vi "DepthProfiling_3D_Core.vi"(5 "BioMAP file path":path=path "", 7 "Params.":variant, 8 "error in (no error)":errorcluster, 9 "Dynamic Params queue":refnum<queue>, 10 "Quit_UserEvent":refnum<user-event>, 11 "ControlQueueRef":variant) -> (0 "error out":errorcluster, 2 "Output":variant)   [LabVIEW 2013]
uses:
  Apps_static/ScanParams_SingleLine.ctl
  ProcessMethods/Binning/BinType.ctl
  Files/BinaryHeader.ctl
  ControlDef/QueueRefs.ctl
  ControlDef/LaserCtrl_Method.ctl
  ControlDef/States-AToF.ctl
  <instrlib>/AnalogDiscSDKLv/VIs/DWF_CtrlQueue.ctl
  <instrlib>/AnalogDiscSDKLv/VIs/DWF_State.ctl
  <instrlib>/ESP300/Public/Data/ESP300_State.ctl
  <instrlib>/DG535/Command/DG535_States.ctl
  Hardware/BNC(QuantumComposers)/BNC_States.ctl
  Hardware/FemtoLaser(Legacy)/Laser_Status.ctl
  Hardware/DAQmx(Legacy)/DAQmx_Status.ctl
  ControlDef/Signal.ctl
  ProcessMethods/SignalAverager/ProcessStates.ctl
  Files/WriterState.ctl
  Files/Signal_Segment.ctl
  ControlDef/ProcessingMode.ctl
  Hardware/EPM2000(Legacy)/EPM2K_Status.ctl
  <instrlib>/AnalogDiscSDKLv/VIs/DWF_Signal.ctl
  ControlDef/SampleRateSelector.ctl
  ImagingMS/DirectImaging_State.ctl
  ImagingMS/Imaging_Params.ctl
  ProcessMethods/BioMapConversion/BioMAPWriterCoreParams.ctl
  <vilib>/Utility/error.llb/DialogType.ctl
  <vilib>/Utility/miscctls.llb/LVRowAndColumnTypeDef.ctl
  <vilib>/picture/picture.llb/imagedata.ctl
  <vilib>/Analysis/baseanly.llb/Mean (DBL).vi
  UI/Autoscale_Y_Single.vi
  <userlib>/_OpenG.lib/comparison/comparison.llb/I32 Changed__ogtk.vi
  ProcessMethods/Binning/SpectrumBinning.vi
  <vilib>/regexp/Match Regular Expression.xnode
  <instrlib>/ESP300/ESP300.lvlib
  <instrlib>/DG535/SRS_DG535_Lib.lvlib
  <userlib>/Utility/ErrorLog_lib.lvlib
  <instrlib>/AnalogDiscSDKLv/AnalogDiscSDKLv.lvlib
  <vilib>/Analysis/NI_AALBase.lvlib
panel:
  out "m/z":dbl=11.0
  in  "Linear/Log":bool
  in  "Integration Width (±Da)":dbl=0.5
  in  "m/z (Da)":dbl=11.0
  in  "BinType":T1=enum."ByMass"
  in  "BinWidth":dbl=0.2 min=0.001
  in  "#Layers":i32=1 caption="LayerAverage#" min=1 max=2000 step=1
  in  "Shot#":i32=1 caption="nth of Shot" min=1 max=65535 step=1
  in  "X--":bool
  in  "X++":bool
  in  "Fullscale X":bool
  in  "Fullscale Y":bool
  in  "Y--":bool
  in  "Y++":bool
  out "Depth Profile":dbl[](graph)
  out "Spectra":cluster{"Array":dbl[], dbl[]}(graph)
  in  "MaxiMass":dbl=300.0 format="%#_13g"
  in  "EnableBinning":bool
  out "Information":string
  in  "AutoScaleZ":bool
  in  "SaveMiddleFile":bool
  in  "Color Scheme":T2(ring)=enum."Rainbow"
  out "#SOL":i32
  out "#EOL":i32
  out "remaining lines":i32
  out "State":T3(ring)
  out "Line#":i32
  in  "Cancel":bool
  in  "Close/Quit":bool
  in  "Peaks of Interest":string[][](table)=[["300", "300"], ["68", ".45"], ["92", ".45"], ["114", ".45"]]
  in  "conv. coeff.":sgl=6553.0
  out "# average":i32
  in  "Start":bool
  out "ImagePreview":dbl[][](graph)
  in  "PeakOI #":i32
  out "MS (Raw)":cluster{"m/z_Array":dbl[], sgl[]}(graph)
  out "Iteration":i32
  out "Export File Path":path caption="Filename"
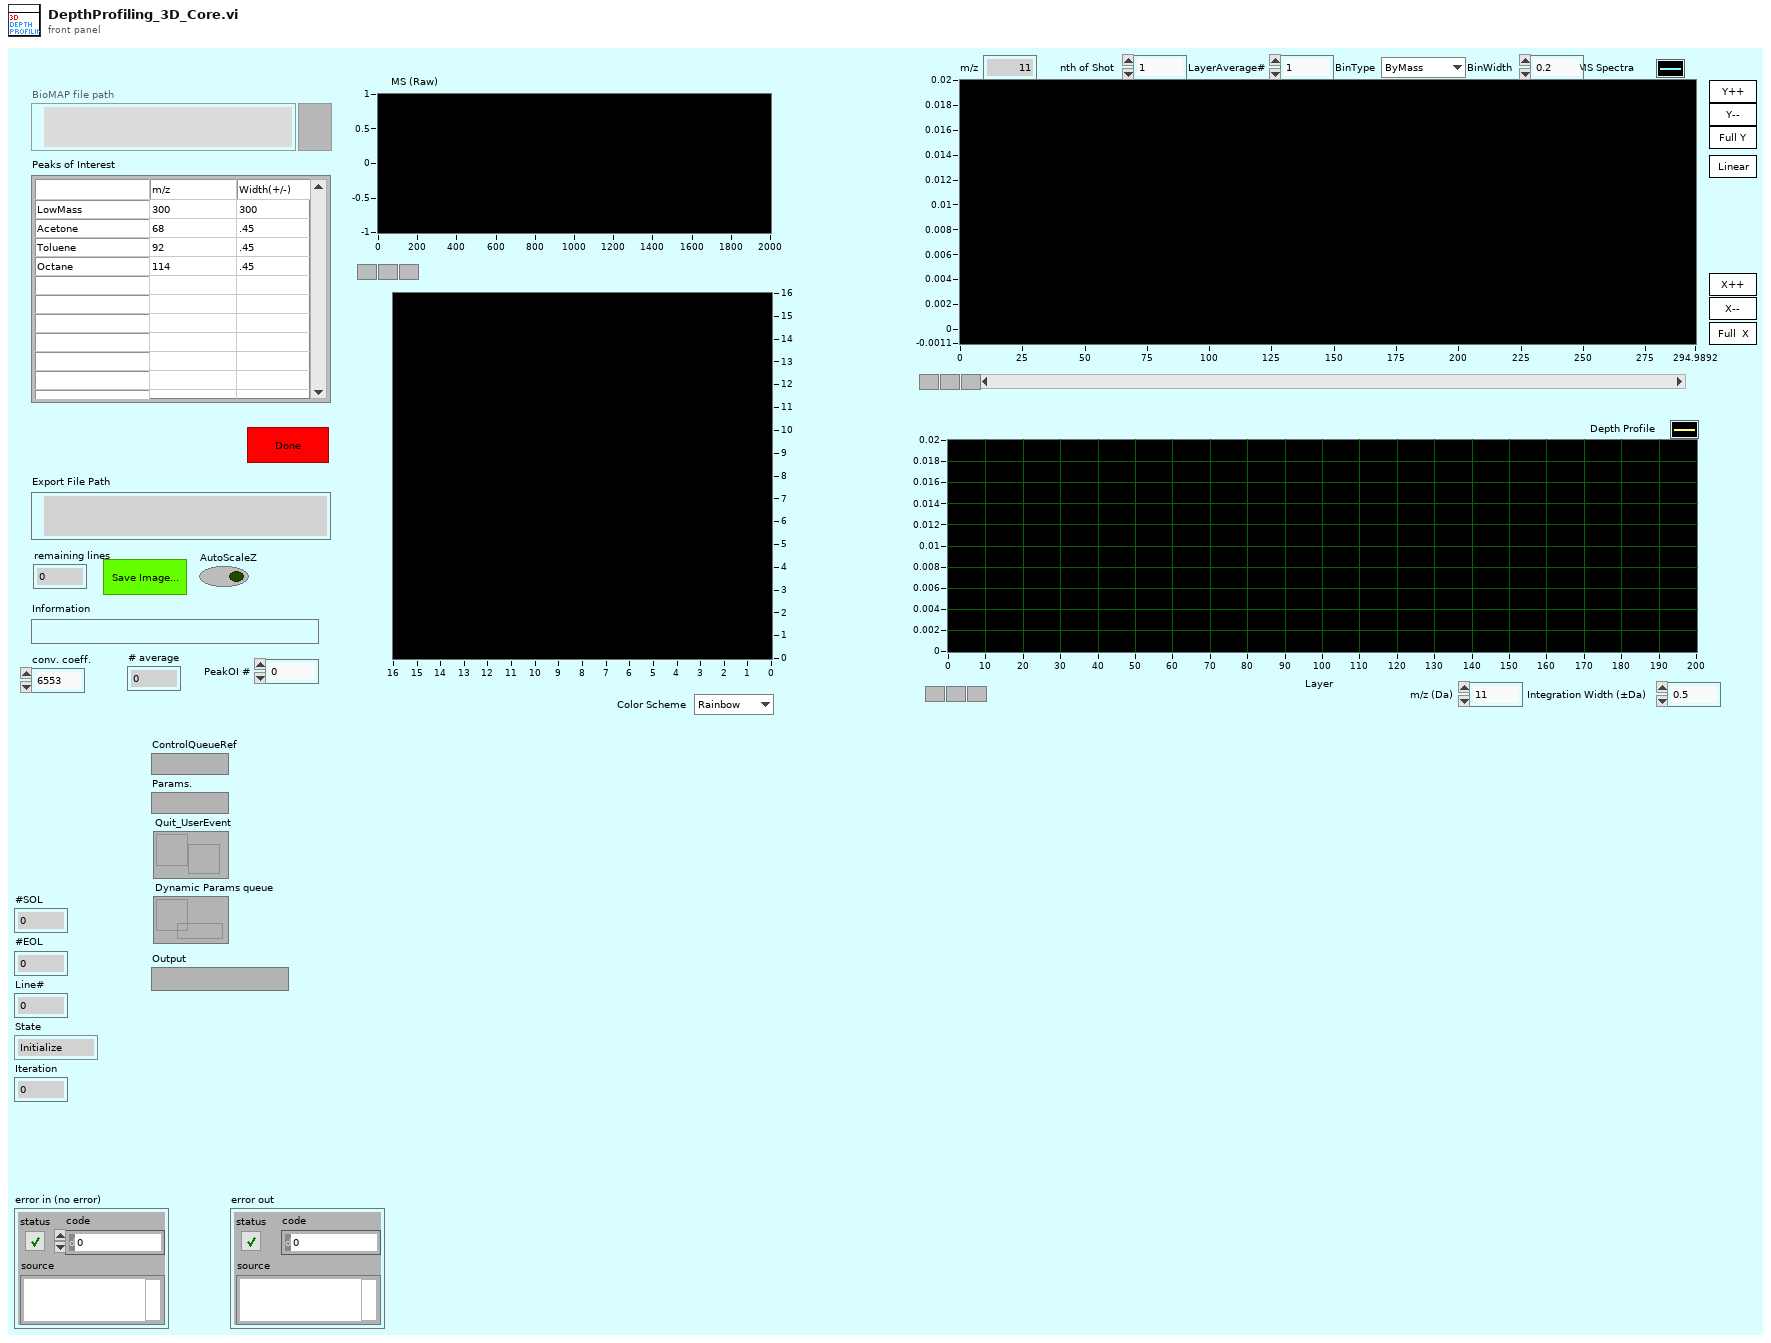
[diagram p1: front panel]
types:
  T1 = typedef "BinType.ctl" = enum16{"ByTime", "ByScreen", "ByMass", "ToUnitMass"}
  T2 = enum16{"Greyscale", "Rainbow", "Jet", "Rainbow_Wh", "Banded", "Seis", "InvertSeis", "Jaisnd", "TBD1"}
  T3 = enum16{"Initialize", "Open", "PrepScanParams", "WaitData", "Flush", "ScanResult", "CheckEndCondition", "Close", "Quit", "Refresh_Image", "Refresh_Profile", "Refresh_Spectra", "Refresh_RawSpectrum", "SaveMiddleFile", "Save_Image", "SetPeakOI"}
  T4 = cluster{"image path":path, "file refnum":refnum<file>}
  T5 = enum8{"Enabled", "Disabled", "Disabled and Grayed Out"}
  T6 = typedef "QueueRefs.ctl" = cluster{"LaserCtrlMethod":T7, "Apps":refnum<queue>, "MainDAQCoreQueue":refnum<queue>, "Micos":refnum<queue>, "ESP300":refnum<queue>, "SMC100":refnum<queue>, "SRS DG535":refnum<queue>, "BNC":refnum<queue>, "SDG_ii":refnum<queue>, "NI-USB_DAQmx":refnum<queue>, "ProcCore_CtrlQueue":refnum<queue>, "WriterCtrl":refnum<queue>, "WriterSIG":refnum<queue>, "Feedback":refnum<queue>, "EPM2000":refnum<queue>, "InfoRef":refnum<vi>, "AppsLock":T8, "ProcCore_SignalQueue":refnum<queue>}
  T7 = typedef "LaserCtrl_Method.ctl" = enum16{"SRS_DG535", "BNC", "SDG_II"}
  T8 = typedef "Semaphore RefNum" = refnum<k1>
  T9 = typedef "ProcessStates.ctl" = enum16{"Initialize", "Normal", "Display", "Write2Buffer", "CalcMzArray", "StartSave", "StopSave", "ConfigChanged", "EndOfLine", "SetFilterParams", "SetGraphsEnable", "SetAcquisitionParams", "ChangeDisplayIncrement", "ChangeRepRate", "SetWriterRef", "Quit", "StartOfLine"}
  T10 = cluster{"Average":i32, "X (Img)":i32, "Y (Img)":i32, "Spectra":sgl[], "Depth":i32, "TickCount":dbl}
  T11 = typedef "BioMAPWriterCoreParams.ctl" = cluster{"File Header":T12, "mzCali.":dbl[], "m/z_Array":dbl[], "SampleRate":T13, "TrigDelay":dbl, "file refnum":refnum<file>, "file path":path, "PeakOI":cluster{"m/z":dbl, "Width(+/-)":dbl}[], "Binning":cluster{"Enable":bool, "BinType":T1, "BinWidth":dbl, "Maximum":dbl, "Minimum":dbl}}
  T12 = typedef "BinaryHeader.ctl" = cluster{"Start Position":dbl[], "StepWidth":dbl[], "Dimension":i32[], "SpecLength":i32}
  T13 = typedef "SampleRateSelector.ctl" = dbl
  T14 = typedef "Imaging_Params.ctl" = cluster{"File Header":T12, "ScanSpeed":dbl, "HighSpeed":dbl, "SampleRate":T13, "Rep.Rate (Hz)":dbl, "TrigDelay":dbl, "mzCali":dbl[], "KeepStill(ms)":u32, "SaveRaw":bool}
  T15 = typedef "DirectImaging_State.ctl" = cluster{"State":enum16{"Initialize", "Open", "PrepScanParams", "WaitData", "Flush", "ScanResult", "CheckEndCondition", "Close", "Quit", "Refresh_Image", "Refresh_Profile", "Refresh_Spectra", "Refresh_RawSpectrum", "SaveMiddleFile", "Save_Image", "SetPeakOI"}, "Para.":variant}
  T16 = cluster{"Save?":bool, "File Header":T12, "Scan#":i32, "ControlRefs":T6, "HighSpeed":dbl, "ScanSpeed":dbl, "SampleRate":T13, "mzCali.":dbl[], "TrigDelay":dbl, "InfoBarRef.":refnum<vi>, "mzArray":dbl[], "SaveRaw":bool, "RepRate":dbl}
  T17 = typedef "LVRowAndColumnTypeDef.ctl" = cluster{"Row":i32, "Column":i32}
  T18 = typedef "DialogType.ctl" = u16
  T19 = typedef "LVPoint32TypeDef.ctl" = cluster{"Horizontal":i32, "Vertical":i32}
  T20 = typedef "LVRectTypeDef.ctl" = cluster{"Left":i16, "Top":i16, "Right":i16, "Bottom":i16}
  T21 = enum16{"open", "replace", "create", "open or create", "replace or create", "replace or create with confirmation"}
  T22 = cluster{"queue out":refnum<queue>, "queue out":refnum<queue>}
  T23 = typedef "Signal.ctl" = cluster{"Command":T9, "Params":variant}
  T24 = typedef "Signal_Segment.ctl" = cluster{"SampleRate":dbl, "TrigDelay":dbl, "SpecLength":dbl, "DAQ_Range":dbl, "Average#":i32, "Position":dbl[], "Spectrum":sgl[], "Calibr.":dbl[], "Pressure":dbl, "Desp_LaserEnergy":dbl, "PI_LaserEnergy":dbl, "Voltages Table":sgl[][], "ProcMode":T25, "Threshold":dbl, "Comment":string, "TickCount":dbl, "Time Stamp":timestamp}
  T25 = typedef "ProcessingMode.ctl" = enum16{"None", "Drop by Threshold", "TDC Simulate", "SetFilter"}
  T26 = typedef "ScanParams_SingleLine.ctl" = cluster{"Line Start":dbl[], "Line End":dbl[], "HighSpeed":dbl, "ScanSpeed":dbl, "KeepStill(ms)":u32, "InstruParams":dbl[]}
  T27 = typedef "imagedata.ctl" = cluster{"image type":i32, "image depth":i32, "image":u8[], "mask":u8[], "colors":u32[], "Rectangle":cluster{"left":i16, "top":i16, "right":i16, "bottom":i16}}
  T28 = cluster{"Rows Per Strip":i32, "Photometric":i32, "Compression Type":i32}
  T29 = cluster{"Average":i32, "X (Img)":i32, "Y (Img)":i32, "Spectra":sgl[], "Depth":i32, "TickCount":dbl}[]
  T30 = typedef "IMAQ Image.ctl" = refnum<image>
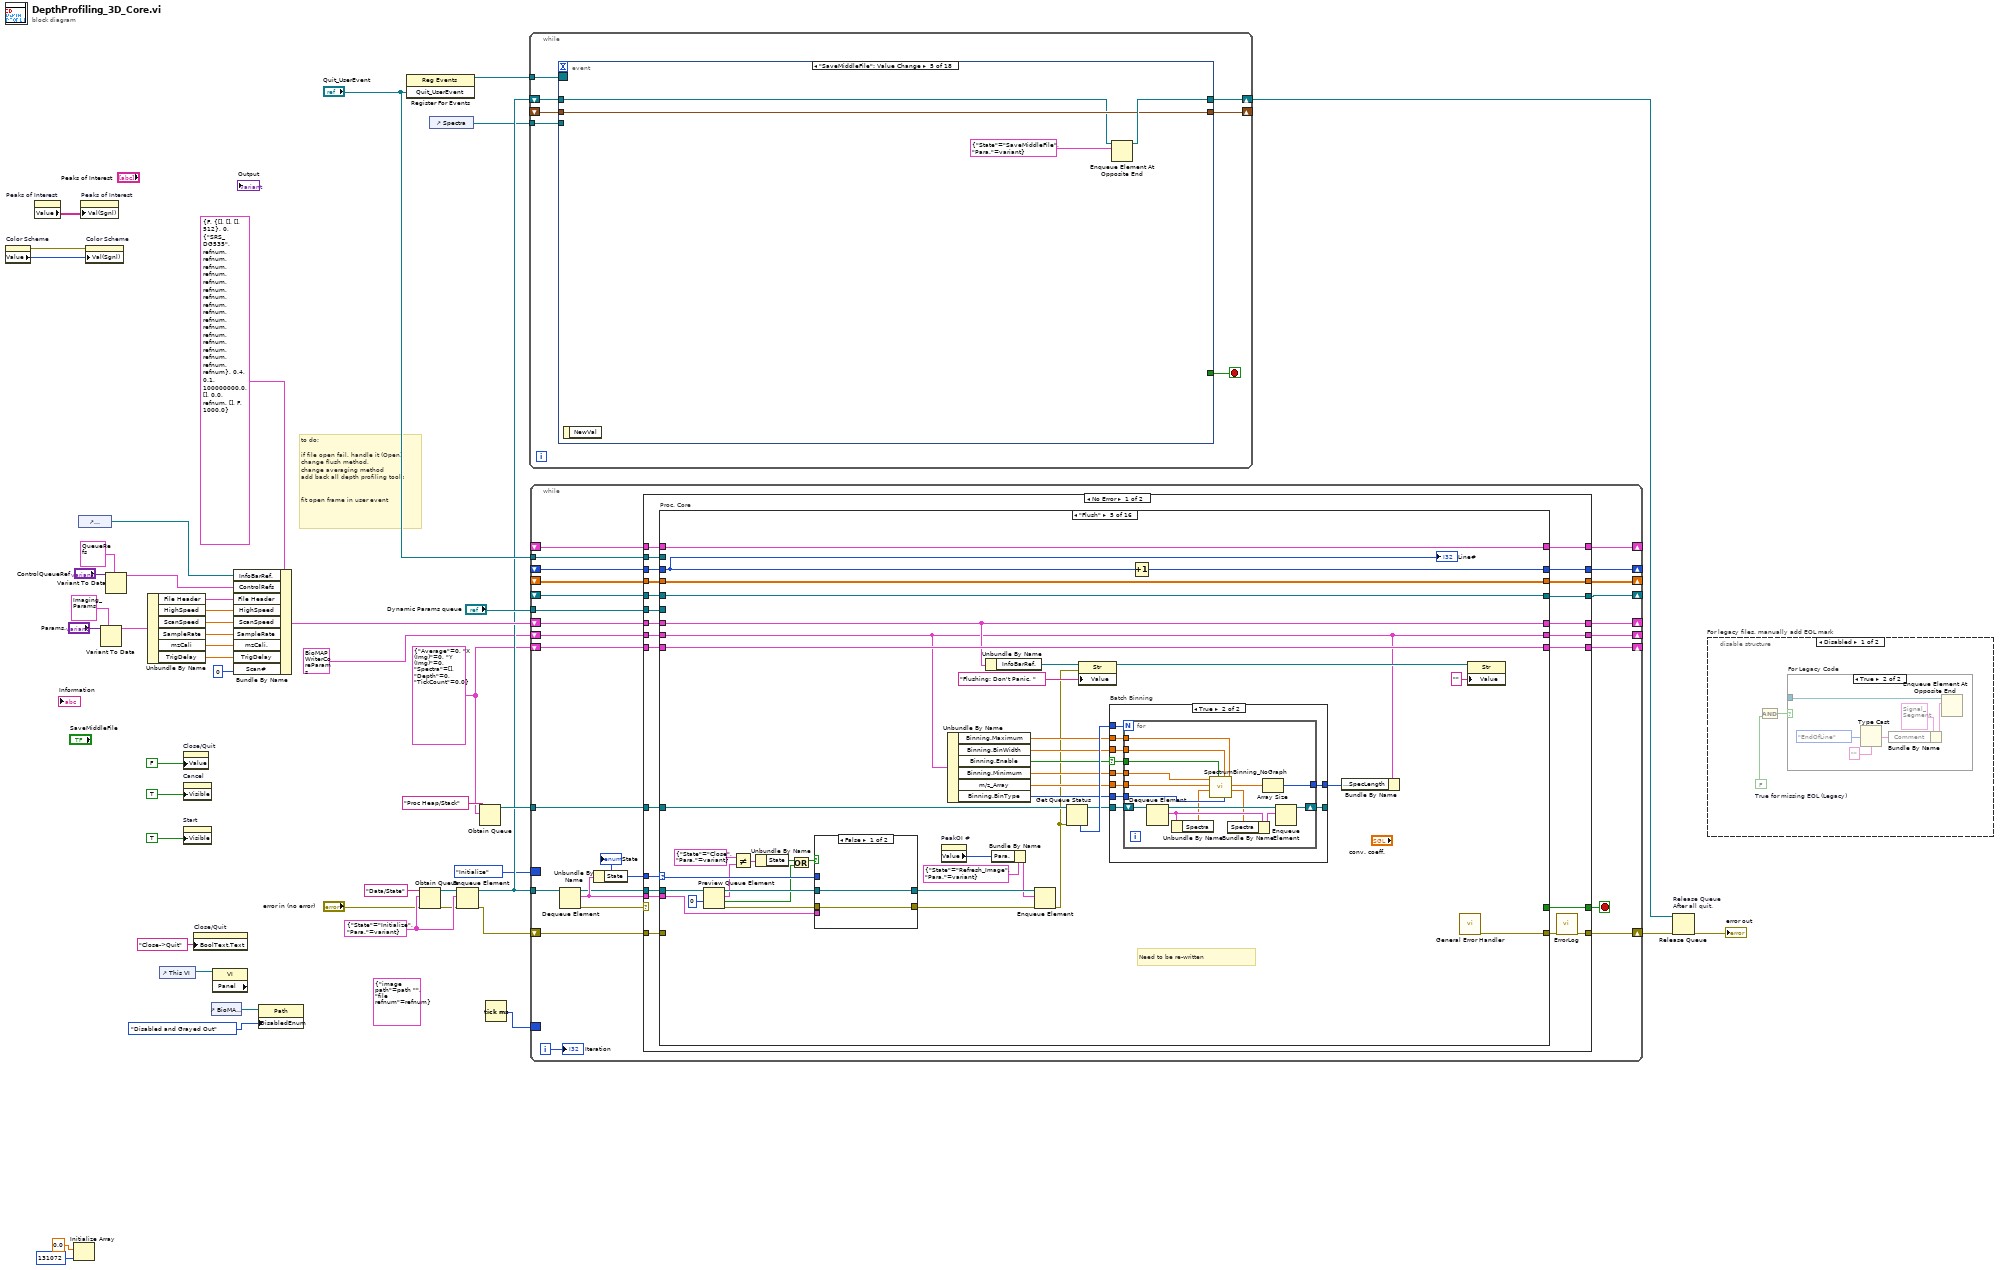
[diagram p0: block diagram]
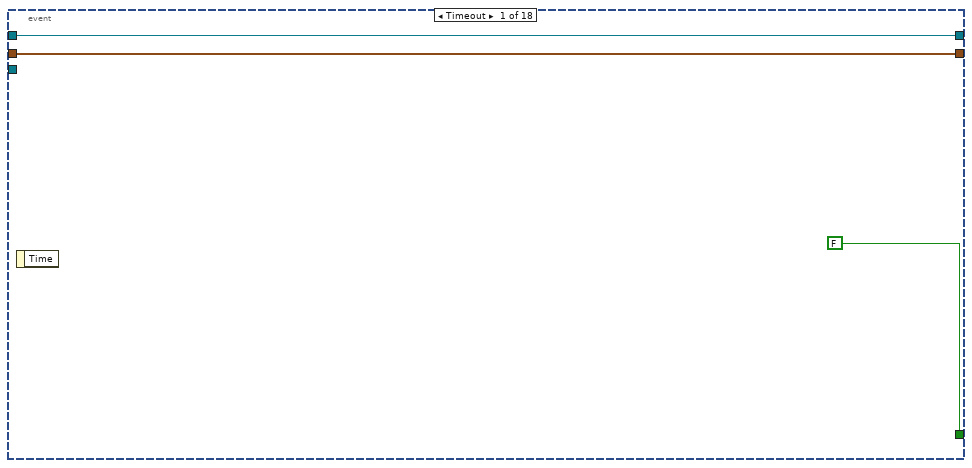
[diagram p4: hidden frame]
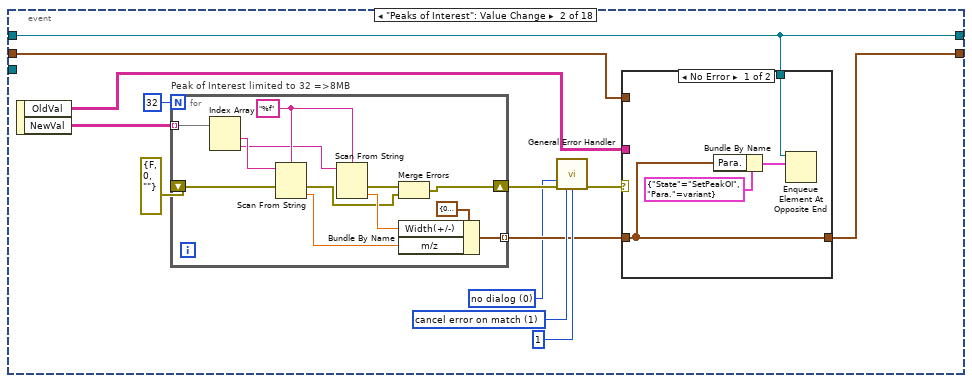
[diagram p5: hidden frame]
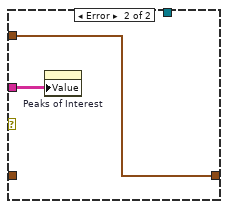
[diagram p6: hidden frame]
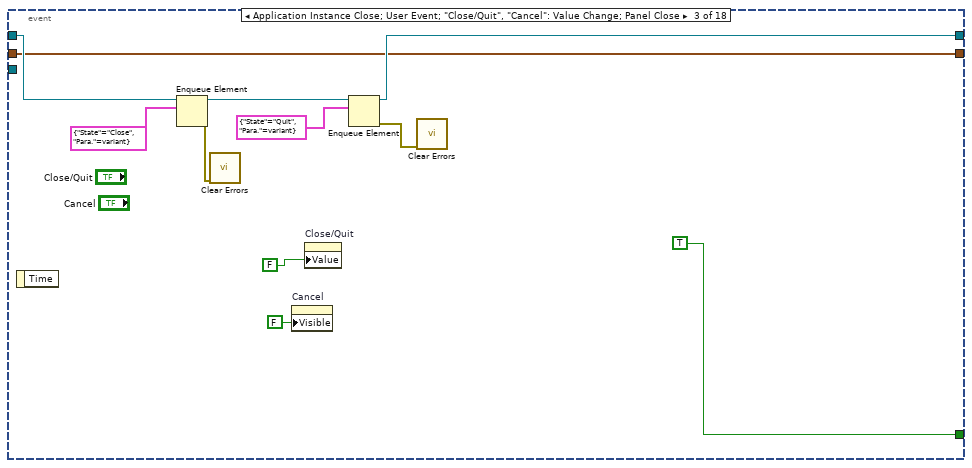
[diagram p7: hidden frame]
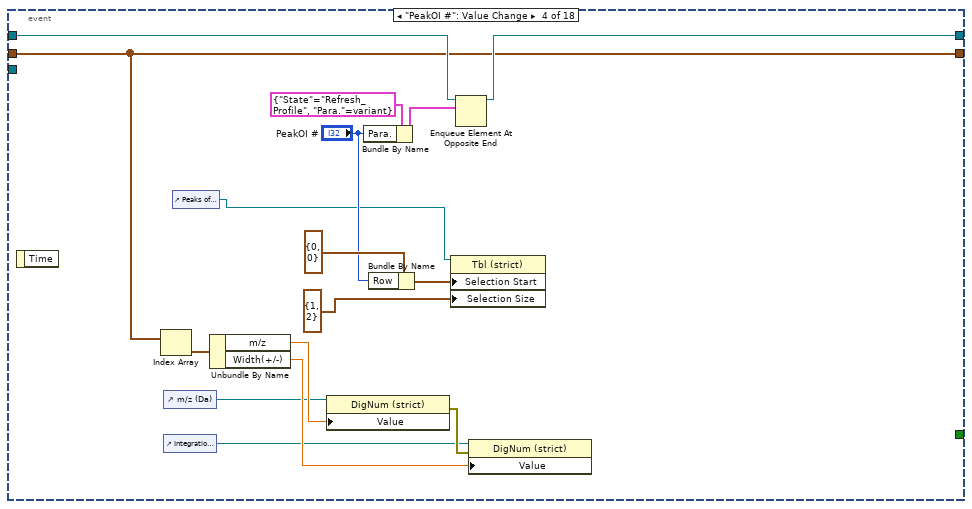
[diagram p8: hidden frame]
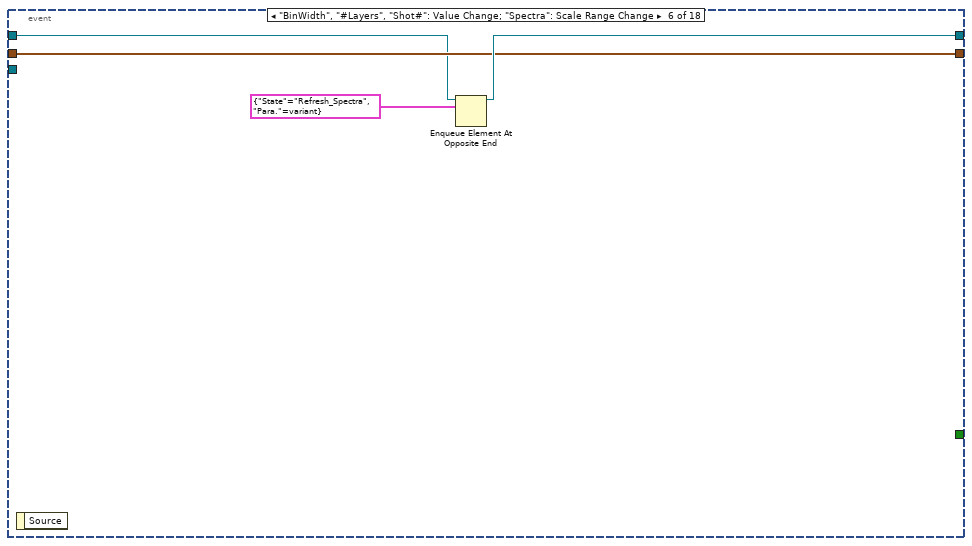
[diagram p9: hidden frame]
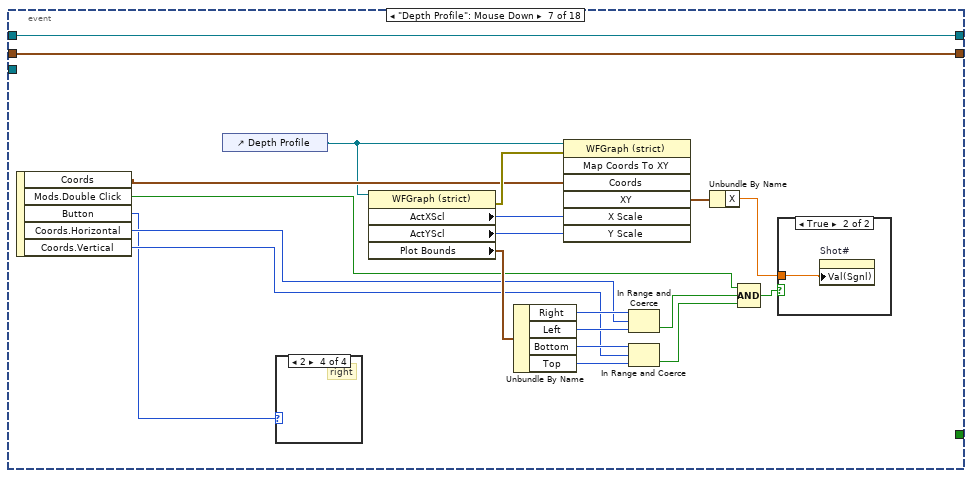
[diagram p10: hidden frame]
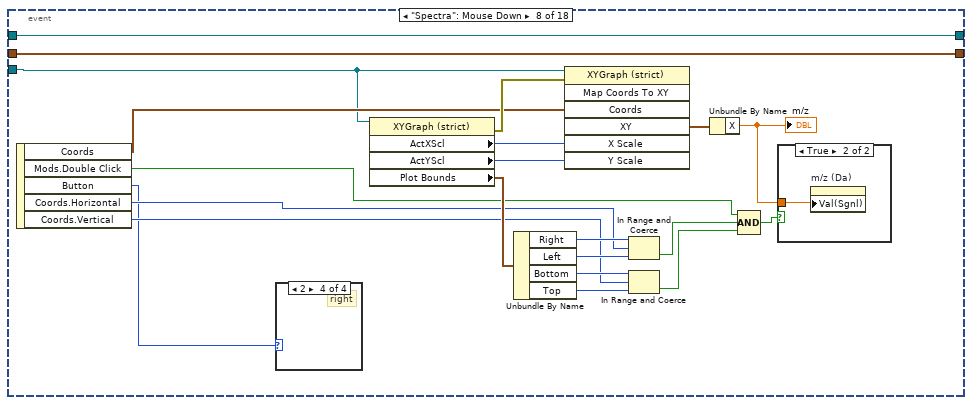
[diagram p15: hidden frame]
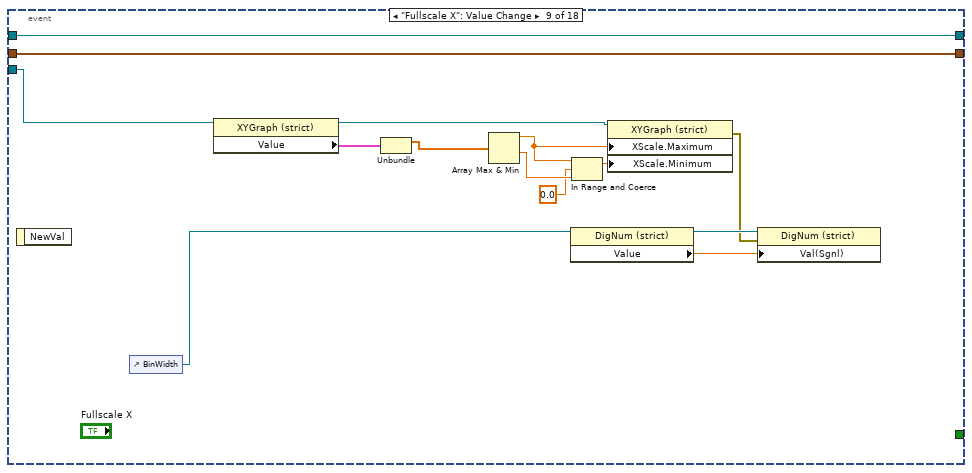
[diagram p20: hidden frame]
diagram:
  (unwired) T4 {"image path"=path "", "file refnum"=refnum} ("output cluster")
  w26 = T10 {"Average"=0, "X (Img)"=0, "Y (Img)"=0, "Spectra"=[], "Depth"=0, "TickCount"=0.0} ("output cluster")
  w38 = T15 {"State"=enum."Initialize", "Para."=variant}
  # "to do;\n\nif file open fail, handle it (Open)\nchange flush method,\nchange averaging method\nadd back all depth profiling tools\n\n\nfit open frame in user event"
  n1 = property on="Color Scheme" class="Enum (strict)"() -> (error out=w2:errorcluster, "Value"=w3:T2)  [unwired: 2 in, 1 out]
  n2 = property on="Peaks of Interest" class="Tbl (strict)"() -> ("Value"=w7:string[][])  [unwired: 2 in, 2 out]
  n3 = Initialize Array(sgl 0.0 ("element"), 131072 ("dimension size")) -> ()  [unwired: 1 out]
  n4 = control-ref of="Information"() -> (w5:refnum<vi>)
  n5 = property on="Peaks of Interest" class="Tbl (strict)"("Val(Sgnl)"=w7) -> ()  [unwired: 2 in, 2 out]
  n6 = property on="Color Scheme" class="Enum (strict)"(error in=w2, "Val(Sgnl)"=w3) -> ()  [unwired: 1 in, 2 out]
  n7 = Variant To Data(type=T14 {"File Header"={"Start Position"=[], "StepWidth"=[], "Dimension"=[], "SpecLength"=0}, "ScanSpeed"=0.0, "HighSpeed"=0.0, "SampleRate"=0.0, "Rep.Rate (Hz)"=0.0, "TrigDelay"=0.0, "mzCali"=[], "KeepStill(ms)"=0, "SaveRaw"=FALSE} ("BeamProfiling_Params"), Variant="Params.") -> (data=w33:T14)  [unwired: 1 in, 1 out]
  n8 = Variant To Data(type=T6 {"LaserCtrlMethod"=enum."SRS_DG535", "Apps"=refnum, "MainDAQCoreQueue"=refnum, "Micos"=refnum, "ESP300"=refnum, "SMC100"=refnum, "SRS DG535"=refnum, "BNC"=refnum, "SDG_ii"=refnum, "NI-USB_DAQmx"=refnum, "ProcCore_CtrlQueue"=refnum, "WriterCtrl"=refnum, "WriterSIG"=refnum, "Feedback"=refnum, "EPM2000"=refnum, "InfoRef"=refnum, "AppsLock"=refnum, "ProcCore_SignalQueue"=refnum} ("ControlRefs"), Variant="ControlQueueRef") -> (data=w13:T6)  [unwired: 1 in, 1 out]
  n9 = Unbundle By Name(w33) -> ("File Header"=w32:T12, "HighSpeed"=w31:dbl, "ScanSpeed"=w30:dbl, "SampleRate"=w28:T13, "mzCali"=w19:dbl[], "TrigDelay"=w18:dbl)
  n10 = control-ref of="This VI"() -> (w17:refnum<vi>)
  n11 = property on="Close/Quit" class="Bool (strict)"("Value"=FALSE) -> ()  [unwired: 2 in, 2 out]
  n12 = property on="Cancel" class="Bool"("Visible"=TRUE) -> ()  [unwired: 2 in, 2 out]
  n13 = property on="Start" class="Bool"("Visible"=TRUE) -> ()  [unwired: 2 in, 2 out]
  n14 = property on="Close/Quit" class="Bool (strict)"("BoolText.Text"="Close->Quit" ("Boolean Text.Text")) -> ()  [unwired: 2 in, 2 out]
  n15 = control-ref of="BioMAP file path"() -> (w12:refnum<vi>)
  n16 = property class="VI" props=["Panel"](reference=w17) -> ()  [unwired: 1 in, 3 out]
  n17 = Bundle By Name(cluster=T16 {"Save?"=FALSE, "File Header"={"Start Position"=[], "StepWidth"=[], "Dimension"=[], "SpecLength"=512}, "Scan#"=0, "ControlRefs"={"LaserCtrlMethod"=enum."SRS_DG535", "Apps"=refnum, "MainDAQCoreQueue"=refnum, "Micos"=refnum, "ESP300"=refnum, "SMC100"=refnum, "SRS DG535"=refnum, "BNC"=refnum, "SDG_ii"=refnum, "NI-USB_DAQmx"=refnum, "ProcCore_CtrlQueue"=refnum, "WriterCtrl"=refnum, "WriterSIG"=refnum, "Feedback"=refnum, "EPM2000"=refnum, "InfoRef"=refnum, "AppsLock"=refnum, "ProcCore_SignalQueue"=refnum}, "HighSpeed"=0.4, "ScanSpeed"=0.1, "SampleRate"=100000000.0, "mzCali."=[], "TrigDelay"=0.0, "InfoBarRef."=refnum, "mzArray"=[], "SaveRaw"=FALSE, "RepRate"=1000.0} ("output cluster"), "InfoBarRef."=w5, "ControlRefs"=w13, "File Header"=w32, "HighSpeed"=w31, "ScanSpeed"=w30, "SampleRate"=w28, "mzCali."=w19, "TrigDelay"=w18, "Scan#"=0) -> (w42:T16)
  n18 = property class="Path"(reference=w12, "DisabledEnum"=T5."Disabled and Grayed Out" ("Disabled")) -> ()  [unwired: 1 in, 2 out]
  n19 = register-events("Quit_UserEvent") -> (reference out=w43:refnum<event-registration>)  [unwired: 2 in, 1 out]
  n20 = Obtain Queue(name (unnamed)="Data/State", element data type=w38, error in (no error)="error in (no error)") -> (queue out=w39:refnum<queue>, error out=w37:errorcluster)  [unwired: 2 in, 1 out]
  n21 = control-ref of="Spectra"() -> (w1:refnum<vi>)
  n22 = Enqueue Element(queue=w39, element=w38, error in (no error)=w37) -> (queue out=w35:refnum<queue>, error out=w27:errorcluster)  [unwired: 1 in, 1 out]
  n23 = Obtain Queue(name (unnamed)="Proc Heap/Stack", element data type=w26) -> (queue out=w48:refnum<queue>)  [unwired: 3 in, 2 out]
  n24 = Tick Count (ms)() -> (millisecond timer value=w25:u32)
  n25 = while {
    tunnel: w43 -> [w53]
    shift-right: [w52] -> w20
    shift-left: w35 -> [w55]
    shift-right: [w51] -> _
    shift-left: _ -> [w50]
    tunnel: w1 -> [w49]
    stop <- w54 stop-if-true
    n26 = event shown="[4] \"SaveMiddleFile\": Value Change" {
      selector: w53 -> [_ _ _ _ _ _ _ _ _ _ _ _ _ _ _ _ _ _]
      dyn-events: _ -> [_ _ _ _ _ _ _ _ _ _ _ _ _ _ _ _ _ _]
      timeout: _ -> [_ _ _ _ _ _ _ _ _ _ _ _ _ _ _ _ _ _]
      tunnel: w55 -> [w57 w59 w97 w113 w117 w121 w145 w167 w182 w185 w192 w210 w228 w250 w279 w290 w313 w345]
      tunnel: [FALSE _ TRUE _ _ _ _ _ _ _ _ _ _ _ _ _ _ _] -> w54
      tunnel: [w57 w59 w93 w114 w119 w123 w145 w167 w182 w185 w192 w210 w228 w250 w279 w290 w308 w344] -> w52
      tunnel: [w56 w64 w92 w104 w118 w122 w144 w166 w181 w184 w191 w209 w227 w249 w278 w287 w310 w343] -> w51
      tunnel: w50 -> [w56 w62 w92 w104 w118 w122 w144 w166 w181 w184 w191 w209 w227 w249 w278 w287 w310 w343]
      tunnel: w49 -> [_ _ _ _ _ _ _ w147 w169 w183 w187 w193 w211 w229 w258 _ _ _]
      event Timeout {
        n27 = event-data() -> ()  [unwired: 1 in, 1 out]
      }
      event "Peaks of Interest": Value Change {
        w60 = T18 0 items=["no dialog", "OK message", "continue or stop message", "OK message + warnings", "continue/stop + warnings"] ("type of dialog (OK msg:1)")
        w65 = 1 items=["no exception", "cancel error on match", "set error on match"] ("[exception action] (none:0)")
        n28 = event-data() -> ("OldVal"=w70:string[][], "NewVal"=w71:string[][])  [unwired: 1 in]
        n29 = for "Peak of Interest limited to 32 =>8MB" {
          N: 32 -> [_]
          tunnel: w71 -> [w83] mode=indexing
          shift-right: [w75] -> w66
          shift-left: errorcluster {"status"=FALSE, "code"=0, "source"=""} ("error IO") -> [w77]
          tunnel: [w76] -> w63 mode=indexing
          w82 = "%f" ("format string")
          n30 = Index Array(array=w83) -> (element #1=w73:string, element #2=w72:string)  [unwired: 2 in]
          n31 = Scan From String(format string=w82, input string=w73, error in=w77) -> (error out=w74:errorcluster, output 1=w79:dbl)  [unwired: 2 in, 2 out]
          n32 = Scan From String(format string=w82, input string=w72) -> (error out=w78:errorcluster, output 1=w80:dbl)  [unwired: 3 in, 2 out]
          n33 = Merge Errors(w78, w74) -> (w75:errorcluster)
          n34 = Bundle By Name(cluster=cluster{"m/z":dbl, "Width(+/-)":dbl} {"m/z"=0.0, "Width(+/-)"=0.0} ("Peak-Of-Interest"), "Width(+/-)"=w80, "m/z"=w79) -> (w76:cluster{"m/z":dbl, "Width(+/-)":dbl})
        }
        n35 = call <vilib>:"General Error Handler.vi"("type of dialog (OK msg:1)"=w60, "error in (no error)"=w66, "[exception action] (none:0)"=w65, "[exception code]"=1) -> ("error out"=w67:errorcluster)  [unwired: 7 in, 4 out]
        n36 = case shown="No Error" w67 {
          tunnel: w70 -> [_ w89]
          tunnel: [w85 w88] -> w64
          tunnel: w63 -> [w85 _]
          tunnel: w62 -> [_ w88]
          tunnel: w59 -> [w84 _]
          frame No Error {
            n37 = Bundle By Name(cluster=T15 {"State"=enum."SetPeakOI", "Para."=variant} ("element"), "Para."=w85) -> (w86:T15)
            n38 = Enqueue Element At Opposite End(queue=w84, element=w86) -> ()  [unwired: 2 in, 3 out]
          }
          frame Error {
            n39 = property on="Peaks of Interest" class="Tbl (strict)"("Value"=w89) -> ()  [unwired: 2 in, 2 out]
          }
        }
      }
      event Application Instance Close; User Event; "Close/Quit", "Cancel": Value Change; Panel Close {
        n40 = event-data() -> ()  [unwired: 1 in, 1 out]
        n41 = Enqueue Element(queue=w97, element=T15 {"State"=enum."Close", "Para."=variant}) -> (queue out=w98:refnum<queue>, error out=w96:errorcluster)  [unwired: 2 in, 1 out]
        n42 = call <vilib>:"Clear Errors.vi"("error in (no error)"=w96) -> ()  [unwired: 6 in, 1 out]
        n43 = property on="Cancel" class="Bool"("Visible"=FALSE) -> ()  [unwired: 2 in, 2 out]
        n44 = property on="Close/Quit" class="Bool (strict)"("Value"=FALSE) -> ()  [unwired: 2 in, 2 out]
        n45 = Enqueue Element(queue=w98, element=T15 {"State"=enum."Quit", "Para."=variant}) -> (queue out=w93:refnum<queue>, error out=w99:errorcluster)  [unwired: 2 in, 1 out]
        n46 = call <vilib>:"Clear Errors.vi"("error in (no error)"=w99) -> ()  [unwired: 6 in, 1 out]
      }
      event "PeakOI #": Value Change {
        n47 = event-data() -> ()  [unwired: 1 in, 1 out]
        n48 = Index Array(array=w104) -> (element=w105:cluster{"m/z":dbl, "Width(+/-)":dbl})  [unwired: 1 in]
        n49 = control-ref of="m/z (Da)"() -> (w102:refnum<vi>)
        n50 = control-ref of="Integration Width (±Da)"() -> (w101:refnum<vi>)
        n51 = control-ref of="Peaks of Interest"() -> (w108:refnum<vi>)
        n52 = Unbundle By Name(w105) -> ("m/z"=w103:dbl, "Width(+/-)"=w106:dbl)
        n53 = property class="DigNum (strict)"(reference=w102, "Value"=w103) -> (error out=w107:errorcluster)  [unwired: 1 in, 1 out]
        n54 = Bundle By Name(cluster=T15 {"State"=enum."Refresh_Profile", "Para."=variant} ("element"), "Para."="PeakOI #") -> (w115:T15)
        n55 = Bundle By Name(cluster=T17 {"Row"=0, "Column"=0} ("Selection Start"), "Row"="PeakOI #") -> (w111:T17)
        n56 = property on="Property Node" class="Tbl (strict)"(reference=w108, "Selection Start"=w111, "Selection Size"=T17 {"Row"=1, "Column"=2}) -> ()  [unwired: 1 in, 2 out]
        n57 = Enqueue Element At Opposite End(queue=w113, element=w115) -> (queue out=w114:refnum<queue>)  [unwired: 2 in, 2 out]
        n58 = property class="DigNum (strict)"(reference=w101, error in=w107, "Value"=w106) -> ()  [unwired: 2 out]
      }
      event "SaveMiddleFile": Value Change {
        n59 = event-data() -> ()  [unwired: 1 in, 1 out]
        n60 = Enqueue Element At Opposite End(queue=w117, element=T15 {"State"=enum."SaveMiddleFile", "Para."=variant}) -> (queue out=w119:refnum<queue>)  [unwired: 2 in, 2 out]
      }
      event "BinWidth", "#Layers", "Shot#": Value Change; "Spectra": Scale Range Change {
        n61 = event-data() -> ()  [unwired: 1 in, 1 out]
        n62 = Enqueue Element At Opposite End(queue=w121, element=T15 {"State"=enum."Refresh_Spectra", "Para."=variant}) -> (queue out=w123:refnum<queue>)  [unwired: 2 in, 2 out]
      }
      event "Depth Profile": Mouse Down {
        n63 = event-data() -> ("Coords"=w126:T19, "Mods.Double Click"=w127:bool, "Button"=w128:u16, "Coords.Horizontal"=w129:i32, "Coords.Vertical"=w130:i32)  [unwired: 1 in]
        n64 = control-ref of="Depth Profile"() -> (w125:refnum<vi>)
        n65 = case shown="2" w128 {
          frame Default {
          }
          frame 3 {
            # "middle"
          }
          frame 1 {
            # "left"
          }
          frame 2 {
            # "right"
          }
        }
        n66 = property on="Property Node" class="WFGraph (strict)"(reference=w125) -> (error out=w131:errorcluster, "ActXScl"=w134:i32, "ActYScl"=w133:i32, "Plot Bounds"=w136:T20)  [unwired: 1 in, 1 out]
        n67 = Unbundle By Name(w136) -> ("Right"=w137:i16, "Left"=w138:i16, "Bottom"=w139:i16, "Top"=w140:i16)
        n68 = invoke on="Invoke Node" class="WFGraph (strict)" method="Map Coords To XY"(reference=w125, error in=w131, "Coords"=w126, "X Scale"=w134, "Y Scale"=w133) -> ("XY"=w132:cluster{"X":dbl, "Y":dbl})  [unwired: 2 in, 6 out]
        n69 = In Range and Coerce(upper limit=w137, x=w129, lower limit=w138) -> (In Range?=w142:bool)  [unwired: 1 out]
        n70 = In Range and Coerce(upper limit=w139, x=w130, lower limit=w140) -> (In Range?=w143:bool)  [unwired: 1 out]
        n71 = Unbundle By Name(w132) -> ("X"=w135:dbl)
        n72 = Compound Arithmetic op=AND(w127, w142, w143) -> (w141:bool)
        n73 = case shown="True" w141 {
          tunnel: w135 -> [_ w146]
          frame False {
          }
          frame True {
            n74 = property on="Shot#" class="DigNum (strict)"("Val(Sgnl)"=w146) -> ()  [unwired: 2 in, 2 out]
          }
        }
      }
      event "Spectra": Mouse Down {
        n75 = event-data() -> ("Coords"=w149:T19, "Mods.Double Click"=w150:bool, "Button"=w151:u16, "Coords.Horizontal"=w152:i32, "Coords.Vertical"=w153:i32)  [unwired: 1 in]
        n76 = case shown="2" w151 {
          frame Default {
          }
          frame 3 {
            # "middle"
          }
          frame 1 {
            # "left"
          }
          frame 2 {
            # "right"
          }
        }
        n77 = property on="Property Node" class="XYGraph (strict)"(reference=w147) -> (error out=w154:errorcluster, "ActXScl"=w157:i32, "ActYScl"=w156:i32, "Plot Bounds"=w158:T20)  [unwired: 1 in, 1 out]
        n78 = Unbundle By Name(w158) -> ("Right"=w159:i16, "Left"=w160:i16, "Bottom"=w161:i16, "Top"=w162:i16)
        n79 = invoke on="Invoke Node" class="XYGraph (strict)" method="Map Coords To XY"(reference=w147, error in=w154, "Coords"=w149, "X Scale"=w157, "Y Scale"=w156) -> ("XY"=w155:cluster{"X":dbl, "Y":dbl})  [unwired: 2 in, 6 out]
        n80 = In Range and Coerce(upper limit=w159, x=w152, lower limit=w160) -> (In Range?=w164:bool)  [unwired: 1 out]
        n81 = In Range and Coerce(upper limit=w161, x=w153, lower limit=w162) -> (In Range?=w165:bool)  [unwired: 1 out]
        n82 = Unbundle By Name(w155) -> ("X"=w148:dbl)
        "m/z" <- w148
        n83 = Compound Arithmetic op=AND(w150, w164, w165) -> (w163:bool)
        n84 = case shown="True" w163 {
          tunnel: w148 -> [_ w168]
          frame False {
          }
          frame True {
            n85 = property on="m/z (Da)" class="DigNum (strict)"("Val(Sgnl)"=w168) -> ()  [unwired: 2 in, 2 out]
          }
        }
      }
      event "Fullscale X": Value Change {
        n86 = event-data() -> ()  [unwired: 1 in, 1 out]
        n87 = control-ref of="BinWidth"() -> (w170:refnum<vi>)
        n88 = property class="XYGraph (strict)"(reference=w169) -> (reference out=w174:refnum<vi>, "Value"=w177:cluster{"Array":dbl[], dbl[]})  [unwired: 1 in, 1 out]
        n89 = Unbundle(w177) -> ("Array"=w176:dbl[])  [unwired: 1 out]
        n90 = Array Max & Min(array=w176) -> (max value=w175:dbl, min value=w180:dbl)  [unwired: 2 out]
        n91 = property class="DigNum (strict)"(reference=w170) -> (reference out=w173:refnum<vi>, "Value"=w172:dbl)  [unwired: 1 in, 1 out]
        n92 = In Range and Coerce(upper limit=w175, x=0.0 ("X Scale.Range:Minimum"), lower limit=w180) -> (coerced(x)=w178:dbl)  [unwired: 1 out]
        n93 = property on="Property Node" class="XYGraph (strict)"(reference=w174, "XScale.Maximum"=w175, "XScale.Minimum"=w178) -> (error out=w171:errorcluster)  [unwired: 1 in, 1 out]
        n94 = property class="DigNum (strict)"(reference=w173, error in=w171, "Val(Sgnl)"=w172) -> ()  [unwired: 2 out]
      }
      event "Fullscale Y": Value Change {
        n95 = event-data() -> ()  [unwired: 1 in, 1 out]
        n96 = call-poly "Autoscale_Y.vi"("GraphRef"=w183) -> ()  [unwired: 11 in]
      }
      event "Linear/Log": Value Change {
        n97 = event-data() -> ()  [unwired: 1 in, 6 out]
        n98 = Select(t=u8 1 ("Y Scale.Mapping Mode"), s="Linear/Log", f=u8 0 ("Y Scale.Mapping Mode")) -> (s? t:f=w190:u8)
        n99 = property on="Property Node" class="XYGraph (strict)"(reference=w187, "YScale.Mapping Mode"=w190) -> ()  [unwired: 1 in, 2 out]
      }
      event "X++": Value Change {
        n100 = event-data() -> ()  [unwired: 1 in, 6 out]
        n101 = property on="Property Node" class="XYGraph (strict)"(reference=w193) -> (reference out=w198:refnum<vi>, "XScale.Maximum"=w199:dbl, "XScale.Minimum"=w200:dbl)  [unwired: 1 in, 1 out]
        n102 = Add(x=w199, y=w200) -> (x+y=w201:dbl)
        n103 = Subtract(x=w199, y=w200) -> (x-y=w204:dbl)
        n104 = control-ref of="BinWidth"() -> (w194:refnum<vi>)
        n105 = Multiply(x=0.5, y=w201) -> (x*y=w205:dbl)
        n106 = Multiply(x=0.25, y=w204) -> (x*y=w206:dbl)
        n107 = Add(x=w205, y=w206) -> (x+y=w207:dbl)
        n108 = Subtract(x=w205, y=w206) -> (x-y=w208:dbl)
        n109 = property class="DigNum (strict)"(reference=w194) -> (reference out=w197:refnum<vi>, "Value"=w196:dbl)  [unwired: 1 in, 1 out]
        n110 = property on="Property Node" class="XYGraph (strict)"(reference=w198, "XScale.Maximum"=w207, "XScale.Minimum"=w208) -> (error out=w195:errorcluster)  [unwired: 1 in, 1 out]
        n111 = property class="DigNum (strict)"(reference=w197, error in=w195, "Val(Sgnl)"=w196) -> ()  [unwired: 2 out]
      }
      event "X--": Value Change {
        n112 = event-data() -> ()  [unwired: 1 in, 6 out]
        n113 = property on="Property Node" class="XYGraph (strict)"(reference=w211) -> (reference out=w216:refnum<vi>, "XScale.Maximum"=w217:dbl, "XScale.Minimum"=w218:dbl)  [unwired: 1 in, 1 out]
        n114 = Add(x=w217, y=w218) -> (x+y=w219:dbl)
        n115 = Subtract(x=w217, y=w218) -> (x-y=w222:dbl)
        n116 = control-ref of="BinWidth"() -> (w212:refnum<vi>)
        n117 = Multiply(x=0.5, y=w219) -> (x*y=w223:dbl)
        n118 = Multiply(x=1.0, y=w222) -> (x*y=w224:dbl)
        n119 = Add(x=w223, y=w224) -> (x+y=w225:dbl)
        n120 = Subtract(x=w223, y=w224) -> (x-y=w226:dbl)
        n121 = property class="DigNum (strict)"(reference=w212) -> (reference out=w215:refnum<vi>, "Value"=w214:dbl)  [unwired: 1 in, 1 out]
        n122 = property on="Property Node" class="XYGraph (strict)"(reference=w216, "XScale.Maximum"=w225, "XScale.Minimum"=w226) -> (error out=w213:errorcluster)  [unwired: 1 in, 1 out]
        n123 = property class="DigNum (strict)"(reference=w215, error in=w213, "Val(Sgnl)"=w214) -> ()  [unwired: 2 out]
      }
      event "Y--": Value Change {
        n124 = event-data() -> ()  [unwired: 1 in, 6 out]
        n125 = property on="Property Node" class="XYGraph (strict)"(reference=w229) -> (reference out=w230:refnum<vi>, "Value"=w231:cluster{"Array":dbl[], dbl[]}, "XScale.Maximum"=w243:dbl, "XScale.Minimum"=w242:dbl, "YScale.Maximum"=w234:dbl, "YScale.Minimum"=w233:dbl)  [unwired: 1 in, 1 out]
        n126 = Unbundle(w231) -> ("Array"=w245:dbl[], w244:dbl[])
        n127 = for {
          tunnel: w244 -> [w252] mode=indexing
          tunnel: w245 -> [w256] mode=indexing
          tunnel: w242 -> [w255]
          tunnel: w243 -> [w254]
          tunnel: [w251] -> w241 mode=indexing
          n128 = In Range and Coerce(upper limit=w254, x=w256, lower limit=w255) -> (In Range?=w253:bool)  [unwired: 1 out]
          n129 = case shown="True" w253 {
            tunnel: w252 -> [_ w257]
            tunnel: [_ w257] -> w251
            frame False {
              (unwired) nan
            }
            frame True {
            }
          }
        }
        n130 = Array Max & Min(array=w241) -> (min value=w235:dbl)  [unwired: 3 out]
        n131 = In Range and Coerce(upper limit=w234, x=w235, lower limit=w233) -> (coerced(x)=w232:dbl)  [unwired: 1 out]
        n132 = Subtract(x=w234, y=w232) -> (x-y=w240:dbl)
        n133 = Subtract(x=w232, y=w233) -> (x-y=w238:dbl)
        n134 = Multiply(x=2.0, y=w240) -> (x*y=w247:dbl)
        n135 = Multiply(x=2.0, y=w238) -> (x*y=w237:dbl)
        n136 = Add(x=w232, y=w247) -> (x+y=w246:dbl)
        n137 = Subtract(x=w232, y=w237) -> (x-y=w236:dbl)
        n138 = property on="Property Node" class="XYGraph (strict)"(reference=w230, "YScale.Maximum"=w246, "YScale.Minimum"=w236) -> ()  [unwired: 1 in, 2 out]
      }
      event "Y++": Value Change {
        n139 = event-data() -> ()  [unwired: 1 in, 6 out]
        n140 = property on="Property Node" class="XYGraph (strict)"(reference=w258) -> (reference out=w259:refnum<vi>, "Value"=w260:cluster{"Array":dbl[], dbl[]}, "XScale.Maximum"=w272:dbl, "XScale.Minimum"=w271:dbl, "YScale.Maximum"=w263:dbl, "YScale.Minimum"=w262:dbl)  [unwired: 1 in, 1 out]
        n141 = Unbundle(w260) -> ("Array"=w274:dbl[], w273:dbl[])
        n142 = for {
          tunnel: w273 -> [w281] mode=indexing
          tunnel: w274 -> [w285] mode=indexing
          tunnel: w271 -> [w284]
          tunnel: w272 -> [w283]
          tunnel: [w280] -> w270 mode=indexing
          n143 = In Range and Coerce(upper limit=w283, x=w285, lower limit=w284) -> (In Range?=w282:bool)  [unwired: 1 out]
          n144 = case shown="True" w282 {
            tunnel: w281 -> [_ w286]
            tunnel: [_ w286] -> w280
            frame False {
              (unwired) nan
            }
            frame True {
            }
          }
        }
        n145 = Array Max & Min(array=w270) -> (min value=w264:dbl)  [unwired: 3 out]
        n146 = In Range and Coerce(upper limit=w263, x=w264, lower limit=w262) -> (coerced(x)=w261:dbl)  [unwired: 1 out]
        n147 = Subtract(x=w263, y=w261) -> (x-y=w269:dbl)
        n148 = Subtract(x=w261, y=w262) -> (x-y=w267:dbl)
        n149 = Multiply(x=0.5, y=w269) -> (x*y=w276:dbl)
        n150 = Multiply(x=0.5, y=w267) -> (x*y=w266:dbl)
        n151 = Add(x=w261, y=w276) -> (x+y=w275:dbl)
        n152 = Subtract(x=w261, y=w266) -> (x-y=w265:dbl)
        n153 = property on="Property Node" class="XYGraph (strict)"(reference=w259, "YScale.Maximum"=w275, "YScale.Minimum"=w265) -> ()  [unwired: 1 in, 2 out]
      }
      event "Color Scheme": Value Change {
        n154 = event-data() -> ()  [unwired: 1 in, 6 out]
        n155 = case shown="\"Rainbow_Wh\"" "Color Scheme" {
          tunnel: [u32[] [0, 65793, 131586, 197379, 263172, 328965, 394758, 460551, 526344, 592137, 657930, 723723, 789516, 855309, 921102, 986895, 1052688, 1118481, 1184274, 1250067, 1315860, 1381653, 1447446, 1513239, 1579032, 1644825, 1710618, 1776411, 1842204, 1907997, 1973790, 2039583, 2105376, 2171169, 2236962, 2302755, 2368548, 2434341, 2500134, 2565927, 2631720, 2697513, 2763306, 2829099, 2894892, 2960685, 3026478, 3092271, 3158064, 3223857, 3289650, 3355443, 3421236, 3487029, 3552822, 3618615, 3684408, 3750201, 3815994, 3881787, 3947580, 4013373, 4079166, 4144959, 4210752, 4276545, 4342338, 4408131, 4473924, 4539717, 4605510, 4671303, 4737096, 4802889, 4868682, 4934475, 5000268, 5066061, 5131854, 5197647, 5263440, 5329233, 5395026, 5460819, 5526612, 5592405, 5658198, 5723991, 5789784, 5855577, 5921370, 5987163, 6052956, 6118749, 6184542, 6250335, 6316128, 6381921, 6447714, 6513507, 6579300, 6645093, 6710886, 6776679, 6842472, 6908265, 6974058, 7039851, 7105644, 7171437, 7237230, 7303023, 7368816, 7434609, 7500402, 7566195, 7631988, 7697781, 7763574, 7829367, 7895160, 7960953, 8026746, 8092539, 8158332, 8224125, 8289918, 8355711, 8421504, 8487297, 8553090, 8618883, 8684676, 8750469, 8816262, 8882055, 8947848, 9013641, 9079434, 9145227, 9211020, 9276813, 9342606, 9408399, 9474192, 9539985, 9605778, 9671571, 9737364, 9803157, 9868950, 9934743, 10000536, 10066329, 10132122, 10197915, 10263708, 10329501, 10395294, 10461087, 10526880, 10592673, 10658466, 10724259, 10790052, 10855845, 10921638, 10987431, 11053224, 11119017, 11184810, 11250603, 11316396, 11382189, 11447982, 11513775, 11579568, 11645361, 11711154, 11776947, 11842740, 11908533, 11974326, 12040119, 12105912, 12171705, 12237498, 12303291, 12369084, 12434877, 12500670, 12566463, 12632256, 12698049, 12763842, 12829635, 12895428, 12961221, 13027014, 13092807, 13158600, 13224393, 13290186, 13355979, 13421772, 13487565, 13553358, 13619151, 13684944, 13750737, 13816530, 13882323, 13948116, 14013909, 14079702, 14145495, 14211288, 14277081, 14342874, 14408667, 14474460, 14540253, 14606046, 14671839, 14737632, 14803425, 14869218, 14935011, 15000804, 15066597, 15132390, 15198183, 15263976, 15329769, 15395562, 15461355, 15527148, 15592941, 15658734, 15724527, 15790320, 15856113, 15921906, 15987699, 16053492, 16119285, 16185078, 16250871, 16316664, 16382457, 16448250, 16514043, 16579836, 16645629, 16711422, 16777215] ("Array") w292 w293 w294 w295 w296 w297 w298 u32[] [0, 262147, 589831, 851978, 1179662, 1441811, 1769495, 2031644, 2359328, 2621478, 2949163, 3276848, 3801147, 4194372, 4456520, 4522061, 4718673, 4849750, 5046363, 5177439, 5242980, 5374056, 5439597, 5505142, 5636218, 5767300, 5636232, 5701773, 5701777, 5701782, 5570714, 5505183, 5505187, 5505192, 5177521, 5111990, 5046458, 4980927, 4587720, 4456652, 4325585, 3932374, 3801306, 3604703, 3014888, 2818284, 2621681, 2359541, 2162938, 1638655, 1048831, 786687, 262399, 255, 1279, 4351, 5631, 6655, 7679, 9983, 11007, 12031, 13311, 16383, 17407, 18687, 21759, 23039, 24063, 25087, 27391, 28415, 29439, 30719, 32767, 34815, 36095, 39167, 40447, 41471, 42495, 44799, 45823, 46847, 48127, 50175, 51199, 55551, 56575, 57855, 58879, 59903, 62207, 63231, 64255, 65535, 65526, 65522, 65518, 65505, 65496, 65492, 65483, 65479, 65475, 65471, 65467, 65458, 65454, 65450, 65437, 65432, 65424, 65415, 65411, 65407, 65403, 65394, 65390, 65386, 65382, 65369, 65364, 65360, 65356, 65343, 65339, 65335, 65326, 65322, 65318, 65305, 65301, 65296, 65292, 65288, 65280, 589568, 851712, 1441536, 1703680, 1965824, 2817792, 3079936, 3407616, 3669760, 4194048, 4456192, 4783872, 5046016, 5897984, 6160128, 6422272, 7274240, 7536384, 7864064, 8126208, 8650496, 8912640, 9240320, 9502464, 10092288, 10616576, 10878720, 11730688, 11992832, 12320512, 12582656, 13106944, 13369088, 13696768, 13958912, 14548736, 14810880, 15924992, 16187136, 16449280, 16776960, 16775680, 16773632, 16772608, 16771328, 16770304, 16768256, 16766976, 16765952, 16762624, 16760576, 16759552, 16757248, 16756224, 16755200, 16753920, 16752896, 16750848, 16749568, 16748544, 16745216, 16744192, 16742144, 16739840, 16738816, 16737792, 16736512, 16734464, 16733440, 16732160, 16731136, 16727808, 16726784, 16725760, 16724736, 16721408, 16720384, 16719104, 16717056, 16716032, 16714752, 16711680, 16711680, 16711680, 16711680, 16711680, 16711680, 16711680, 16711680, 16711680, 16711680, 16711680, 16711680, 16711680, 16711680, 16711680, 16711680, 16711680, 16711680, 15527148, 15592941, 15658734, 15724527, 15790320, 15856113, 15921906, 15987699, 16053492, 16119285, 16185078, 16250871, 16316664, 16382457, 16448250, 16514043, 16579836, 16645629, 16711422, 16777215] ("appended array")] -> w288
          frame "Greyscale", Default {
          }
          frame "Rainbow" {
            w292 = u32[] [0, 0, 12517567, 12320960, 12189888, 12058817, 11927746, 11731139, 11600067, 9175197, 9044125, 11141318, 11010246, 10813639, 10682568, 10551497, 10354890, 10223818, 10092747, 7930019, 7798948, 9633997, 9502926, 9306319, 9175248, 9044176, 8847569, 8716498, 8585427, 6750377, 6619306, 8126677, 7995606, 7798999, 7667927, 7536856, 7340249, 7209178, 7078106, 5505199, 5374128, 6619357, 6488285, 6291678, 6160607, 6029536, 5832929, 5701857, 5570786, 4325557, 4194486, 5112036, 4980965, 4784358, 4653287, 4522215, 4325608, 4194537, 4063466, 3080380, 3014844, 3604716, 3408109, 3277038, 3277038, 3145966, 3014895, 2818288, 2687217, 2556145, 1900738, 1769666, 2097396, 1900789, 1769717, 1638646, 1507575, 1310968, 1179896, 1048825, 721096, 590024, 590075, 393468, 262397, 131326, 255, 1791, 3327, 4863, 5068, 6348, 9471, 11007, 12543, 14079, 15615, 17151, 18687, 20223, 17612, 18636, 25087, 26623, 28159, 29695, 31231, 32767, 34303, 35839, 29900, 31180, 40447, 41983, 43775, 45311, 46847, 48383, 49919, 51455, 42444, 43724, 56063, 57599, 59135, 60671, 62207, 63743, 65535, 65528, 52418, 52413, 65510, 65504, 65498, 65492, 65486, 65480, 65474, 65468, 52369, 52364, 65449, 65443, 65437, 65431, 65425, 65419, 65413, 65407, 52321, 52316, 65389, 65383, 65377, 65371, 65364, 65358, 65352, 65346, 52272, 52267, 65328, 65322, 65316, 65310, 65304, 65298, 65292, 65286, 52224, 314368, 851712, 1244928, 1638144, 2031360, 2424576, 2817792, 3211008, 3604224, 3197952, 3525632, 4783872, 5177088, 5635840, 6029056, 6422272, 6815488, 7208704, 7601920, 6409216, 6736896, 6736896, 8781568, 9174784, 9568000, 9961216, 10354432, 10747648, 11206400, 11599616, 9554944, 9882624, 12779264, 13172480, 13565696, 13958912, 14352128, 14745344, 15138560, 15531776, 12766208, 13093888, 16776960, 16775170, 16773637, 16771847, 16770314, 16768780, 16766991, 16765457, 13411088, 13409810, 16760601, 16758812, 16757278, 16755745, 16753955, 16752422, 16750888, 16749099, 13398052, 13396774, 16744243, 16742704, 16741166, 16739884, 16738345, 16736807, 16735269, 16733730, 13385753, 13384728, 16729371, 16727833, 16726295, 16725012, 16723474, 16721936, 16720397, 16718859, 13373959, 13372677, 16714500, 16712962, 16777215]  # Color table (Rainbow-striped)
          }
          frame "Jet" {
            w293 = u32[] [127, 131, 135, 139, 143, 147, 151, 155, 159, 163, 167, 171, 175, 179, 183, 187, 191, 195, 199, 203, 207, 211, 215, 219, 223, 227, 231, 235, 239, 243, 247, 251, 255, 1279, 2303, 3327, 4351, 5375, 6399, 7423, 8447, 9471, 10495, 11519, 12543, 13567, 14591, 15615, 16639, 17663, 18687, 19711, 20735, 21759, 22783, 23807, 24831, 25855, 26879, 27903, 28927, 29951, 30975, 31999, 33023, 34047, 35071, 36095, 37119, 38143, 39167, 40191, 41215, 42239, 43263, 44287, 45311, 46335, 47359, 48383, 49407, 50431, 51455, 52479, 53503, 54527, 55551, 56575, 57599, 58623, 59647, 60671, 61695, 62719, 63743, 64767, 131069, 393209, 655349, 917489, 1179629, 1441769, 1703909, 1966049, 2228189, 2490329, 2752469, 3014609, 3276749, 3538889, 3801029, 4063169, 4325309, 4587449, 4849589, 5111729, 5373869, 5636009, 5898149, 6160289, 6422429, 6684569, 6946709, 7208849, 7470989, 7733129, 7995269, 8257409, 8519549, 8781689, 9043829, 9305969, 9568109, 9830249, 10092389, 10354529, 10616669, 10878809, 11140949, 11403089, 11665229, 11927369, 12189509, 12451649, 12713789, 12975929, 13238069, 13500209, 13762349, 14024489, 14286629, 14548769, 14810909, 15073049, 15335189, 15597329, 15859469, 16121609, 16383749, 16645889, 16776192, 16775168, 16774144, 16773120, 16772096, 16771072, 16770048, 16769024, 16768000, 16766976, 16765952, 16764928, 16763904, 16762880, 16761856, 16760832, 16759808, 16758784, 16757760, 16756736, 16755712, 16754688, 16753664, 16752640, 16751616, 16750592, 16749568, 16748544, 16747520, 16746496, 16745472, 16744448, 16743424, 16742400, 16741376, 16740352, 16739328, 16738304, 16737280, 16736256, 16735232, 16734208, 16733184, 16732160, 16731136, 16730112, 16729088, 16728064, 16727040, 16726016, 16724992, 16723968, 16722944, 16721920, 16720896, 16719872, 16718848, 16717824, 16716800, 16715776, 16714752, 16713728, 16712704, 16711680, 16449536, 16187392, 15925248, 15663104, 15400960, 15138816, 14876672, 14614528, 14352384, 14090240, 13828096, 13565952, 13303808, 13041664, 12779520, 12517376, 12255232, 11993088, 11730944, 11468800, 11206656, 10944512, 10682368, 10420224, 10158080, 9895936, 9633792, 9371648, 9109504, 8847360, 8585216, 8323072]  # Jet(256)
          }
          frame "Rainbow_Wh" {
            w294 = u32[] [0, 262147, 589831, 851978, 1179662, 1441811, 1769495, 2031644, 2359328, 2621478, 2949163, 3276848, 3801147, 4194372, 4456520, 4522061, 4718673, 4849750, 5046363, 5177439, 5242980, 5374056, 5439597, 5505142, 5636218, 5767300, 5636232, 5701773, 5701777, 5701782, 5570714, 5505183, 5505187, 5505192, 5177521, 5111990, 5046458, 4980927, 4587720, 4456652, 4325585, 3932374, 3801306, 3604703, 3014888, 2818284, 2621681, 2359541, 2162938, 1638655, 1048831, 786687, 262399, 255, 1279, 4351, 5631, 6655, 7679, 9983, 11007, 12031, 13311, 16383, 17407, 18687, 21759, 23039, 24063, 25087, 27391, 28415, 29439, 30719, 32767, 34815, 36095, 39167, 40447, 41471, 42495, 44799, 45823, 46847, 48127, 50175, 51199, 55551, 56575, 57855, 58879, 59903, 62207, 63231, 64255, 65535, 65526, 65522, 65518, 65505, 65496, 65492, 65483, 65479, 65475, 65471, 65467, 65458, 65454, 65450, 65437, 65432, 65424, 65415, 65411, 65407, 65403, 65394, 65390, 65386, 65382, 65369, 65364, 65360, 65356, 65343, 65339, 65335, 65326, 65322, 65318, 65305, 65301, 65296, 65292, 65288, 65280, 589568, 851712, 1441536, 1703680, 1965824, 2817792, 3079936, 3407616, 3669760, 4194048, 4456192, 4783872, 5046016, 5897984, 6160128, 6422272, 7274240, 7536384, 7864064, 8126208, 8650496, 8912640, 9240320, 9502464, 10092288, 10616576, 10878720, 11730688, 11992832, 12320512, 12582656, 13106944, 13369088, 13696768, 13958912, 14548736, 14810880, 15924992, 16187136, 16449280, 16776960, 16775680, 16773632, 16772608, 16771328, 16770304, 16768256, 16766976, 16765952, 16762624, 16760576, 16759552, 16757248, 16756224, 16755200, 16753920, 16752896, 16750848, 16749568, 16748544, 16745216, 16744192, 16742144, 16739840, 16738816, 16737792, 16736512, 16734464, 16733440, 16732160, 16731136, 16727808, 16726784, 16725760, 16724736, 16721408, 16720384, 16719104, 16717056, 16716032, 16714752, 16711680, 16711680, 16711680, 16711680, 16711680, 16711680, 16711680, 16711680, 16711680, 16711680, 16711680, 16711680, 16711680, 16711680, 16711680, 16711680, 16711680, 16711680, 16777215, 16777215, 16777215, 16777215, 16777215, 16777215, 16777215, 16777215, 16777215, 16777215, 16777215, 16777215, 16777215, 16777215, 16777215, 16777215, 16777215, 16777215, 16777215, 16777215]  # Rainbow+White (237)
          }
          frame "Banded" {
            w295 = u32[] [6750846, 7013765, 7211659, 7409807, 7476371, 7411604, 7214997, 7017621, 6754453, 6490776, 6358685, 6226596, 6226092, 6226101, 6226109, 6227140, 6293961, 6296012, 6297806, 6233806, 5906635, 5512904, 4922053, 4199363, 3542212, 2950855, 2425550, 2031830, 1638622, 1376741, 1246954, 1314285, 1447407, 1975278, 2305771, 2372838, 2242272, 1783259, 1323992, 799448, 340956, 79842, 15849, 17905, 151543, 481786, 1009148, 1667324, 2193914, 2457333, 2523375, 2260968, 1801698, 1276895, 752607, 360418, 99816, 36335, 38390, 237307, 632574, 1158654, 1815550, 2275323, 2537717, 2471662, 2208487, 1683426, 1158879, 634847, 308451, 48362, 50673, 52728, 316924, 777214, 1302782, 1893373, 2352122, 2548212, 2481645, 2087398, 1628129, 1038303, 580576, 254949, 60394, 62189, 129520, 392688, 851694, 1441515, 2031078, 2423264, 2552791, 2419661, 2024898, 1499321, 974770, 516526, 190124, 60844, 62635, 129707, 458153, 982695, 1572516, 2161825, 2488475, 2552211, 2353800, 1893501, 1368177, 843623, 451166, 124759, 61010, 62797, 195401, 589383, 1113670, 1703494, 2227014, 2553410, 2551868, 2287665, 1827364, 1302294, 974603, 1040900, 1239041, 1699840, 2291200, 3013379, 3866121, 4783634, 5635611, 6355746, 6878502, 7073317, 7071521, 7004697, 6938385, 7069705, 7398403, 7858688, 8515840, 9172992, 9894916, 10550795, 11140627, 11599132, 11926051, 12055590, 11988261, 11855391, 11723032, 11788047, 11984904, 12510467, 13101824, 13759232, 14416129, 15006981, 15400460, 15728149, 15858974, 15857956, 15659558, 15395620, 15065886, 14736150, 14669582, 14800391, 15128322, 15587840, 16047616, 16441345, 16637958, 16703246, 16702743, 16570656, 16307237, 15846438, 15385379, 14924316, 14660116, 14658828, 14854661, 15182337, 15641344, 16100352, 16493826, 16690440, 16690192, 16690201, 16492833, 16163878, 15703078, 15242018, 14846235, 14647058, 14645003, 14840068, 15232513, 15690496, 16083200, 16410371, 16541193, 16541202, 16410139, 16213282, 15818789, 15292709, 14831136, 14434840, 14169616, 14166537, 14360579, 14686208, 15077888, 15404288, 15600132, 15665675, 15536665, 15342119, 15015986, 14558008, 14033211, 13507643, 13047097, 12848439, 12781367, 12911162, 13107263, 13303877, 13500748, 13501524, 13371996, 13177188, 12851050, 12393581, 11869549, 11278955, 10753384, 10293092, 9963875, 9765987, 9765220, 9764967, 9699434, 9634157, 9372526, 9111662, 8719469, 8261738]  # Banded(256)
          }
          frame "Seis" {
            w296 = u32[] [11206656, 11403264, 11599872, 11796480, 11993088, 12189696, 12386304, 12582912, 12779520, 12976128, 13172736, 13369344, 13565952, 13762560, 13959168, 14155776, 14352384, 14548992, 14745600, 14942208, 15138816, 15335424, 15532032, 15728640, 15925248, 16121856, 16318464, 16515072, 16711680, 16712448, 16713216, 16713984, 16714752, 16715520, 16716288, 16717056, 16717824, 16718592, 16719360, 16720128, 16720896, 16721664, 16722432, 16723200, 16723968, 16724736, 16725504, 16726272, 16727040, 16727808, 16728576, 16729344, 16730112, 16730880, 16731648, 16732416, 16733184, 16733952, 16734720, 16735488, 16736256, 16737024, 16737792, 16738560, 16739328, 16740096, 16740864, 16741632, 16742400, 16743168, 16743936, 16744448, 16745216, 16745984, 16746752, 16747520, 16748288, 16749056, 16749824, 16750592, 16751360, 16752128, 16752896, 16753664, 16754432, 16755200, 16755968, 16756736, 16757504, 16758272, 16759040, 16759808, 16760576, 16761344, 16762112, 16762880, 16763648, 16764416, 16765184, 16765952, 16766720, 16767488, 16768256, 16769024, 16769792, 16770560, 16771328, 16772096, 16772864, 16773632, 16774400, 16775168, 16775936, 16776704, 16776960, 16776960, 16776960, 16776960, 16776960, 16776960, 16776960, 16776960, 16776960, 16776960, 16776960, 16776960, 16776960, 16776960, 16776960, 16776960, 16776960, 16776960, 16776960, 16776960, 16776960, 16776960, 16776960, 16776960, 16776960, 16776960, 16776960, 16776960, 16645888, 16252673, 15924994, 15531779, 15138565, 14745350, 14352135, 14024456, 13631241, 13238026, 12844811, 12451596, 12123917, 11730702, 11337487, 10944272, 10551057, 10223378, 9830163, 9436948, 9043733, 8650518, 8322840, 7929625, 7536410, 7143195, 6749980, 6422301, 6029086, 5766944, 5570083, 5373222, 5176617, 4979756, 4717615, 4520753, 4324148, 4127287, 3930682, 3733821, 3471679, 3274818, 3078213, 2881352, 2684747, 2487886, 2225744, 2028883, 1832278, 1635417, 1438556, 1241950, 979553, 782948, 586087, 389482, 192620, 60784, 59509, 57979, 56704, 55173, 53642, 52367, 50836, 49305, 48030, 46499, 44968, 43694, 42163, 40888, 39357, 37826, 36551, 35020, 33489, 32214, 30684, 29409, 27878, 26347, 25072, 23541, 22010, 20735, 19965, 19195, 18426, 17912, 17142, 16372, 15603, 14833, 14319, 13549, 12780, 12010, 11240, 10726, 9957, 9187, 8417, 7647, 7134, 6364, 5594, 4824, 4055, 3541, 2771, 2001, 1232, 462]  # Seis(256)
          }
          frame "InvertSeis" {
            w297 = u32[] [462, 1232, 2001, 2771, 3541, 4055, 4824, 5594, 6364, 7134, 7647, 8417, 9187, 9957, 10726, 11240, 12010, 12780, 13549, 14319, 14833, 15603, 16372, 17142, 17912, 18426, 19195, 19965, 20735, 22010, 23541, 25072, 26347, 27878, 29409, 30684, 32214, 33489, 35020, 36551, 37826, 39357, 40888, 42163, 43694, 44968, 46499, 48030, 49305, 50836, 52367, 53642, 55173, 56704, 57979, 59509, 60784, 192620, 389482, 586087, 782948, 979553, 1241950, 1438556, 1635417, 1832278, 2028883, 2225744, 2487886, 2684747, 2881352, 3078213, 3274818, 3471679, 3733821, 3930682, 4127287, 4324148, 4520753, 4717615, 4979756, 5176617, 5373222, 5570083, 5766944, 6029086, 6422301, 6749980, 7143195, 7536410, 7929625, 8322840, 8650518, 9043733, 9436948, 9830163, 10223378, 10551057, 10944272, 11337487, 11730702, 12123917, 12451596, 12844811, 13238026, 13631241, 14024456, 14352135, 14745350, 15138565, 15531779, 15924994, 16252673, 16645888, 16776960, 16776960, 16776960, 16776960, 16776960, 16776960, 16776960, 16776960, 16776960, 16776960, 16776960, 16776960, 16776960, 16776960, 16776960, 16776960, 16776960, 16776960, 16776960, 16776960, 16776960, 16776960, 16776960, 16776960, 16776960, 16776960, 16776960, 16776960, 16776704, 16775936, 16775168, 16774400, 16773632, 16772864, 16772096, 16771328, 16770560, 16769792, 16769024, 16768256, 16767488, 16766720, 16765952, 16765184, 16764416, 16763648, 16762880, 16762112, 16761344, 16760576, 16759808, 16759040, 16758272, 16757504, 16756736, 16755968, 16755200, 16754432, 16753664, 16752896, 16752128, 16751360, 16750592, 16749824, 16749056, 16748288, 16747520, 16746752, 16745984, 16745216, 16744448, 16743936, 16743168, 16742400, 16741632, 16740864, 16740096, 16739328, 16738560, 16737792, 16737024, 16736256, 16735488, 16734720, 16733952, 16733184, 16732416, 16731648, 16730880, 16730112, 16729344, 16728576, 16727808, 16727040, 16726272, 16725504, 16724736, 16723968, 16723200, 16722432, 16721664, 16720896, 16720128, 16719360, 16718592, 16717824, 16717056, 16716288, 16715520, 16714752, 16713984, 16713216, 16712448, 16711680, 16515072, 16318464, 16121856, 15925248, 15728640, 15532032, 15335424, 15138816, 14942208, 14745600, 14548992, 14352384, 14155776, 13959168, 13762560, 13565952, 13369344, 13172736, 12976128, 12779520, 12582912, 12386304, 12189696, 11993088, 11796480, 11599872, 11403264, 11206656]  # InvertSeis(256)
          }
          frame "Jaisnd" {
            w298 = u32[] [3014783, 2949253, 2818187, 2621584, 2424982, 2228379, 2031776, 1769637, 1507497, 1245358, 917682, 655542, 327866, 190, 1218, 2757, 4041, 5580, 6863, 8402, 9941, 11480, 12763, 14301, 15840, 17378, 18916, 20198, 21736, 23274, 24556, 25837, 27375, 28656, 29938, 31219, 32500, 33781, 35062, 36343, 37368, 38649, 39673, 40698, 41723, 42747, 43772, 44796, 45821, 46589, 47613, 48381, 49406, 50174, 50942, 51710, 52478, 53502, 54270, 55038, 55806, 122110, 122878, 188926, 189695, 255999, 322303, 388607, 454911, 521215, 587519, 653823, 720127, 851966, 917499, 1048568, 1114101, 1245170, 1376239, 1441772, 1572841, 1703910, 1900515, 2031584, 2162653, 2293722, 2490327, 2621396, 2818001, 3014606, 3145676, 3342281, 3538886, 3735492, 3932097, 4194239, 4390845, 4587451, 4849593, 5046199, 5308341, 5570484, 5832626, 6029233, 6356912, 6619055, 6881199, 7143343, 7471022, 7733166, 8060847, 8388527, 8716208, 9043890, 9371571, 9764789, 10158007, 10485690, 10878908, 11337664, 11730884, 12189640, 12648397, 13172690, 13762520, 14352351, 15073256, 15990772, 16515059, 16318437, 16121818, 15990737, 15925192, 15859648, 15794105, 15794098, 15728556, 15728549, 15728543, 15794074, 15794068, 15859598, 15925129, 15925124, 15990655, 16056186, 16121717, 16252785, 16318316, 16383848, 16514916, 16580448, 16711515, 16776792, 16776276, 16775760, 16775244, 16774985, 16774469, 16773954, 16773439, 16772923, 16772408, 16771893, 16771378, 16770863, 16770093, 16769578, 16769063, 16768549, 16767778, 16767264, 16766750, 16765980, 16765465, 16764695, 16763925, 16763412, 16762642, 16761872, 16761103, 16760333, 16759564, 16758538, 16757769, 16757000, 16755975, 16755206, 16754181, 16753156, 16752131, 16751106, 16684546, 16683521, 16682497, 16681472, 16680192, 16679168, 16677888, 16676608, 16675328, 16674048, 16672768, 16671488, 16604672, 16603136, 16601856, 16600320, 16533248, 16531712, 16464640, 16463104, 16396032, 16328960, 16327168, 16260096, 16192768, 16125696, 16058368, 15991296, 15925252, 15859722, 15728657, 15663128, 15532062, 15466533, 15335467, 15204401, 15073335, 14942269, 14811203, 14680137, 14483535, 14352468, 14155865, 13959262, 13762659, 13566056, 13369452, 13172848, 12910708, 12714103, 12451962, 12189821, 11927679, 11665537, 11403394, 11075716, 10813572, 10485893, 10158212, 9830532, 9437315, 9109633, 8716415, 8323197]  # Jaisnd(256)
          }
          frame "TBD1" {
          }
        }
        n156 = property on="ImagePreview" class="IntGraph (strict)"("Color Table"=w288) -> ()  [unwired: 2 in, 2 out]
      }
      event "Start": Value Change {
        # "must check file exisance"
        n157 = event-data() -> ()  [unwired: 1 in, 1 out]
        n158 = while {
          tunnel: [w317] -> w304
          stop <- w318 stop-if-true
          n159 = Not A Number/Path/Refnum?(number/path/refnum="BioMAP file path") -> (NaN/Path/Refnum?=w315:bool)
          n160 = feedback #1(path "" ("selected path")) -> (w322:path)
          n161 = case shown="True" w315 {
            tunnel: w322 -> [_ w331]
            tunnel: [w324 w330] -> w320
            tunnel: [FALSE ("cancelled") w329] -> w319
            tunnel: "BioMAP file path" -> [w324 _]
            frame False {
            }
            frame True {
              n162 = Strip Path(path=w331) -> (stripped path=w326:path, name=w327:string)
              n163 = call "File Dialog2"("start path"=w326, "default name"=w327, "pattern (all files)"="*.img", "pattern label"="BioMAP Analyze v7.5") -> ("selected path"=w330:path, "cancelled"=w329:bool)  [unwired: 8 in, 2 out]
            }
          }
          n164 = case shown="True" w319 {
            tunnel: w320 -> [w334 _]
            tunnel: [w334 w342] -> w321
            tunnel: w322 -> [_ w342]
            tunnel: [w333 w341] -> w318
            tunnel: [w334 path "" ("selected path")] -> w317
            frame False {
              w332 = FALSE  # legacy
              n165 = Compound Arithmetic op=AND(invert w332, TRUE) -> (w333:bool)
              "Export File Path" <- w334
            }
            frame True {
              n166 = Two Button Dialog(message="No file saving?", 1:"No saving" ("F button name (\"Cancel\")"), 2:"Set filenare" ("T button name (\"OK\")")) -> (T button?=w336:bool)
              n167 = Not(x=w336) -> (.not. x?=w341:bool)
            }
          }
          n168 = feedback-in #1(w321) -> ()
        }
        n169 = property on="Start" class="Bool"("Visible"=FALSE) -> ()  [unwired: 2 in, 2 out]
        n170 = Bundle By Name(cluster=T15 {"State"=enum."SetPeakOI", "Para."=variant} ("element"), "Para."=w310) -> (w311:T15)
        n171 = Enqueue Element At Opposite End(queue=w313, element=w311) -> (queue out=w307:refnum<queue>)  [unwired: 2 in, 2 out]
        n172 = control-ref of="MaxiMass"() -> (w303:refnum<vi>)
        n173 = control-ref of="EnableBinning"() -> (w300:refnum<vi>)
        n174 = Bundle By Name(cluster=T15 {"State"=enum."Open", "Para."=variant} ("element"), "Para."=w304) -> (w305:T15)
        n175 = property class="DigNum (strict)"(reference=w303, "Visible"=FALSE) -> ()  [unwired: 1 in, 2 out]
        n176 = property class="Bool (strict)"(reference=w300, "Visible"=FALSE) -> ()  [unwired: 1 in, 2 out]
        n177 = Enqueue Element At Opposite End(queue=w307, element=w305) -> (queue out=w308:refnum<queue>)  [unwired: 2 in, 2 out]
      }
      event "m/z (Da)", "Integration Width (±Da)": Value Change {
        n178 = event-data() -> ()  [unwired: 1 in, 1 out]
        n179 = Enqueue Element(queue=w345, element=T15 {"State"=enum."Refresh_Profile", "Para."=variant}) -> (queue out=w344:refnum<queue>)  [unwired: 2 in, 2 out]
      }
    }
  }
  n180 = while {
    shift-right: [w365] -> _
    shift-left: w42 -> [w372]
    shift-right: [w364] -> _
    shift-left: _ -> [w371]
    tunnel: w35 -> [w370]
    tunnel: w48 -> [w368]
    tunnel: "Dynamic Params queue" -> [w361]
    shift-right: [w362] -> _
    shift-left: _ -> [w360]
    shift-right: [w359] -> _
    shift-left: _ -> [w358]
    tunnel: "Quit_UserEvent" -> [w357]
    shift-right: [w355] -> w22
    shift-left: w27 -> [w356]
    shift-right: [w351] -> _
    shift-left: w26 -> [w354]
    shift-right: [w352] -> _
    shift-left: T11 {"File Header"={"Start Position"=[], "StepWidth"=[], "Dimension"=[], "SpecLength"=0}, "mzCali."=[], "m/z_Array"=[], "SampleRate"=500000000.0, "TrigDelay"=0.0, "file refnum"=refnum, "file path"=path "", "PeakOI"=[], "Binning"={"Enable"=FALSE, "BinType"=enum."ByTime", "BinWidth"=0.0, "Maximum"=0.0, "Minimum"=0.0}} ("output cluster") -> [w353]
    border: w25 -> [_]
    border: ProcessStates."Initialize" -> [_]
    shift-right: [w348] -> _
    shift-left: _ -> [w347]
    i -> [w349]
    stop <- w363 stop-if-true
    n181 = Dequeue Element(queue=w370) -> (queue out=w366:refnum<queue>, element=w367:T15, error out=w369:errorcluster)  [unwired: 2 in, 1 out]
    n182 = Unbundle By Name(w367) -> ("State"=w350:T3)
    "State" <- w350
    n183 = case shown="No Error" w369 {
      tunnel: w372 -> [w396 w1338]
      tunnel: [w395 w1338] -> w365
      tunnel: w371 -> [w394 w1337]
      tunnel: [w393 w1337] -> w364
      tunnel: w368 -> [w392 _]
      tunnel: w350 -> [w391 _]
      tunnel: w367 -> [w390 _]
      tunnel: w366 -> [w389 _]
      tunnel: [w388 TRUE] -> w363
      tunnel: [w387 w1335] -> w362
      tunnel: w361 -> [w386 _]
      tunnel: w360 -> [w385 w1335]
      tunnel: [w384 w1334] -> w359
      tunnel: w358 -> [w383 w1334]
      tunnel: w357 -> [w382 _]
      tunnel: w356 -> [w381 w1333]
      tunnel: [w375 w1333] -> w355
      tunnel: w354 -> [w380 w1331]
      tunnel: w353 -> [w379 w1332]
      tunnel: [w378 w1332] -> w352
      tunnel: [w377 w1331] -> w351
      tunnel: [w374 w1330] -> w348
      tunnel: w347 -> [w373 w1330]
      frame No Error {
        n184 = case "Proc. Core" shown="\"Flush\"" w391 {
          selector: w391 -> [_ w495 w522 _ w759 w807 _ _ _ _ _ _ _ _ _ _]
          tunnel: w396 -> [w413 w432 w536 w579 w738 w812 w820 w994 w1016 w1047 w1049 w1078 w1123 w1133 w1318 w1329]
          tunnel: [w399 w502 w518 w580 w738 w812 w820 w994 w1016 w1047 w1049 w1078 w1123 w1133 w1318 w1329] -> w395
          tunnel: [w419 0 w516 w614 w749 w804 w837 w998 w1015 w1046 w1064 w1092 w1122 w1179 w1309 w1328] -> w393
          tunnel: w394 -> [w419 _ w516 w614 w748 w804 w837 w998 w1015 w1046 w1064 w1092 w1122 w1179 w1309 w1328]
          tunnel: w392 -> [_ _ _ w610 w727 _ _ _ w1013 _ _ _ _ _ _ _]
          tunnel: w390 -> [_ w458 w524 w612 w760 w808 _ _ _ w1038 _ _ _ w1172 w1317 _]
          tunnel: w389 -> [_ w496 w525 w613 w761 w809 w822 _ _ _ _ _ _ _ _ _]
          tunnel: [_ _ _ _ _ _ _ _ TRUE _ _ _ _ _ _ _] -> w388
          tunnel: [w418 w481 w520 w611 w756 w806 w834 w992 w1012 w1041 w1063 w1091 w1121 w1175 w1310 w1327] -> w387
          tunnel: w386 -> [_ _ w527 _ _ _ _ _ w1005 _ _ _ _ _ _ _]
          tunnel: w385 -> [w418 _ w520 w611 w756 w806 w834 w992 w1012 w1041 w1063 w1091 w1121 w1175 w1310 w1327]
          tunnel: [w417 w491 w517 w594 w758 w805 w833 w984 w1011 w1045 w1062 w1090 w1120 w1178 w1308 w1326] -> w384
          tunnel: w383 -> [w417 _ w517 w594 w758 w805 w833 w984 w1011 w1045 w1062 w1090 w1120 w1178 w1308 w1326]
          tunnel: w382 -> [_ _ _ _ _ _ _ _ w1010 _ _ _ _ _ _ _]
          tunnel: w381 -> [w416 _ w515 w609 _ w803 w832 w978 w1000 w1044 w1061 w1089 w1119 w1177 w1319 w1325]
          tunnel: [w416 w469 w514 w609 w755 w803 w832 w978 w1001 w1044 w1061 w1089 w1119 w1177 w1319 w1325] -> w376
          tunnel: w380 -> [w402 w433 w512 w606 w757 w801 w831 w979 w1003 w1042 w1059 w1087 w1118 w1176 w1321 w1323]
          tunnel: w379 -> [w415 w467 w513 w581 w726 w802 w819 w980 w1004 w1043 w1060 w1088 w1107 w1132 w1315 w1324]
          tunnel: [w414 w470 w513 w581 w726 w802 w819 w980 w1004 w1043 w1060 w1088 w1107 w1132 w1320 w1324] -> w378
          tunnel: [w402 w433 w512 w607 w757 w801 w831 w979 w1003 w1042 w1059 w1087 w1118 w1176 w1321 w1323] -> w377
          tunnel: [w397 w434 w511 w578 w721 w800 w813 w976 w999 w1020 w1051 w1079 w1106 w1130 w1307 w1322] -> w374
          tunnel: w373 -> [w397 _ w511 w578 w721 w800 w813 w976 w999 w1020 w1051 w1079 w1106 w1130 w1307 w1322]
          frame "Initialize" {
            w398 = 0  # Scan#, should not be reset to 0 in "open", for 3D imaging.
            n185 = Unbundle By Name(w413) -> ("File Header.SpecLength"=w409:i32, "File Header"=w407:T12, "mzCali."=w412:dbl[], "SampleRate"=w410:T13, "TrigDelay"=w411:dbl)
            n186 = disable-structure shown="Disabled" {
              frame Disabled {
                w420 = u32[] [0, 0, 12517567, 12320960, 12189888, 12058817, 11927746, 11731139, 11600067, 9175197, 9044125, 11141318, 11010246, 10813639, 10682568, 10551497, 10354890, 10223818, 10092747, 7930019, 7798948, 9633997, 9502926, 9306319, 9175248, 9044176, 8847569, 8716498, 8585427, 6750377, 6619306, 8126677, 7995606, 7798999, 7667927, 7536856, 7340249, 7209178, 7078106, 5505199, 5374128, 6619357, 6488285, 6291678, 6160607, 6029536, 5832929, 5701857, 5570786, 4325557, 4194486, 5112036, 4980965, 4784358, 4653287, 4522215, 4325608, 4194537, 4063466, 3080380, 3014844, 3604716, 3408109, 3277038, 3277038, 3145966, 3014895, 2818288, 2687217, 2556145, 1900738, 1769666, 2097396, 1900789, 1769717, 1638646, 1507575, 1310968, 1179896, 1048825, 721096, 590024, 590075, 393468, 262397, 131326, 255, 1791, 3327, 4863, 5068, 6348, 9471, 11007, 12543, 14079, 15615, 17151, 18687, 20223, 17612, 18636, 25087, 26623, 28159, 29695, 31231, 32767, 34303, 35839, 29900, 31180, 40447, 41983, 43775, 45311, 46847, 48383, 49919, 51455, 42444, 43724, 56063, 57599, 59135, 60671, 62207, 63743, 65535, 65528, 52418, 52413, 65510, 65504, 65498, 65492, 65486, 65480, 65474, 65468, 52369, 52364, 65449, 65443, 65437, 65431, 65425, 65419, 65413, 65407, 52321, 52316, 65389, 65383, 65377, 65371, 65364, 65358, 65352, 65346, 52272, 52267, 65328, 65322, 65316, 65310, 65304, 65298, 65292, 65286, 52224, 314368, 851712, 1244928, 1638144, 2031360, 2424576, 2817792, 3211008, 3604224, 3197952, 3525632, 4783872, 5177088, 5635840, 6029056, 6422272, 6815488, 7208704, 7601920, 6409216, 6736896, 6736896, 8781568, 9174784, 9568000, 9961216, 10354432, 10747648, 11206400, 11599616, 9554944, 9882624, 12779264, 13172480, 13565696, 13958912, 14352128, 14745344, 15138560, 15531776, 12766208, 13093888, 16776960, 16775170, 16773637, 16771847, 16770314, 16768780, 16766991, 16765457, 13411088, 13409810, 16760601, 16758812, 16757278, 16755745, 16753955, 16752422, 16750888, 16749099, 13398052, 13396774, 16744243, 16742704, 16741166, 16739884, 16738345, 16736807, 16735269, 16733730, 13385753, 13384728, 16729371, 16727833, 16726295, 16725012, 16723474, 16721936, 16720397, 16718859, 13373959, 13372677, 16714500, 16712962, 16777215]  # Color table (Rainbow-striped)
                # "Probably to be deleted"
                n187 = property on="ImagePreview" class="IntGraph (strict)"("Color Table"=w420) -> ()  [unwired: 2 in, 2 out]
              }
              frame Enabled {
              }
            }
            n188 = in-place "Compensate error in float-point number calculation" {
              n189 = in-place-cluster #2(w407) -> ("StepWidth"=w421:dbl[], "Start Position"=w426:dbl[])
              n190 = Index Array(array=w421) -> (element=w425:dbl)  [unwired: 1 in]
              n191 = Multiply(x=w425, y=0.001) -> (x*y=w423:dbl)
              n192 = in-place {
                in-place-border: w423 -> [w428]
                n193 = in-place-array #3(w426, 0) -> (w429:dbl)
                n194 = Subtract(x=w429, y=w428) -> (x-y=w430:dbl)
                n195 = in-place-array #3(w430) -> (w427:dbl[])  [unwired: 1 out]
              }
              n196 = in-place-cluster #2("StepWidth"=w421, "Start Position"=w427) -> (w406:T12)
            }
            n197 = Subtract "Gage DAQ does not always gives same length spectrum"(x=w409, y=64) -> (x-y=w400:i32)
            n198 = call "CalcMzArray.vi"("TrigDelay"=w411, "Sample Rate"=w410, "Depth"=w400, "mzCali. (a/b/c)"=w412) -> ("mzArray"=w401:dbl[])  [unwired: 7 in]
            n199 = Bundle By Name(cluster=w413, "Scan#"=w398) -> (w399:T16)
            n200 = Bundle By Name(cluster=w415, "Binning.BinType"=BinType."ByMass", "Binning.BinWidth"=0.1, "Binning.Minimum"=0.0, "File Header.SpecLength"=w400, "m/z_Array"=w401, "File Header"=w406, "mzCali."=w412, "SampleRate"=w410, "TrigDelay"=w411) -> (w414:T11)
          }
          frame "Open" {
            (unwired) T22 {"queue out"=refnum, "queue out"=refnum} ("output cluster")
            w476 = "ActionCallBack" ("name (unnamed)")
            # "Save Header + MzArray first.\nIn case of program crash, \nBioMAP v3.8+ will load partial file just fine."
            # "8192x32KB*4 = 1GB\n!! attention:\nshould be big"
            n201 = Increment(x=w495) -> (x+1=w497:T3)
            n202 = Unbundle By Name(w432) -> ("File Header.SpecLength"=w444:i32, "File Header.Dimension"=w438:i32[], "mzCali."=w440:dbl[], "SampleRate"=w441:T13, "TrigDelay"=w442:dbl)
            n203 = Bundle By Name(cluster=w458, "State"=w497) -> (w498:T15)
            n204 = Unbundle By Name(w458) -> ("Para."=w457:variant)
            n205 = Enqueue Element(queue=w496, element=w498) -> ()  [unwired: 2 in, 3 out]
            n206 = Variant To Data(type=path "" ("selected path"), Variant=w457) -> (data=w449:path, error out=w453:errorcluster)  [unwired: 1 in]
            n207 = call "CalcMzArray.vi"("TrigDelay"=w442, "Sample Rate"=w441, "Depth"=w444, "mzCali. (a/b/c)"=w440) -> ("mzArray"=w443:dbl[])  [unwired: 7 in]
            n208 = Initialize Array(sgl 0.0 ("element"), w444) -> (w436:sgl[])
            n209 = Bundle By Name(cluster=w432, "mzArray"=w443) -> (w431:T16)
            n210 = Open/Create/Replace File(file path (use dialog)=w449, error in=w453, operation (0:open)=T21."create", access (0:read/write)=enum16{"read/write", "read-only", "write-only"}."write-only") -> (refnum out=w447:refnum<file>, error out=w451:errorcluster)  [unwired: 2 in, 1 out]
            n211 = Obtain Queue(max queue size (-1, unlimited)=4096, name (unnamed)="BeamProfiling_Buffer", element data type=T24 {"SampleRate"=0.0, "TrigDelay"=0.0, "SpecLength"=0.0, "DAQ_Range"=0.0, "Average#"=0, "Position"=[], "Spectrum"=[], "Calibr."=[], "Pressure"=0.0, "Desp_LaserEnergy"=0.0, "PI_LaserEnergy"=0.0, "Voltages Table"=[], "ProcMode"=enum."None", "Threshold"=0.0, "Comment"="", "TickCount"=0.0, "Time Stamp"=timestamp(0 s since 1904-01-01)} ("Signal Segment")) -> (queue out=w491:refnum<queue>, error out=w490:errorcluster)  [unwired: 2 in, 1 out]
            n212 = Obtain Queue(name (unnamed)=w476, element data type=w476) -> (queue out=w473:refnum<queue>)  [unwired: 3 in, 2 out]
            n213 = Index Array(array=w438, index=2) -> ()  [unwired: 1 out]
            n214 = Bundle By Name(cluster=w433, "Spectra"=w436) -> (w435:T10)
            n215 = case shown="Error" w451 {
              selector: w451 -> [_ w510]
              tunnel: [_ w510] -> w450
              tunnel: w449 -> [w504 w506]
              tunnel: [w504 w506] -> w448
              tunnel: w447 -> [w503 w505]
              tunnel: [w503 w505] -> w446
              frame No Error {
              }
              frame Error {
                n216 = Two Button Dialog(message="Error when create image file.", 1:"No saving" ("F button name (\"Cancel\")"), 2:"Ignore" ("T button name (\"OK\")")) -> ()  [unwired: 1 out]
              }
            }
            n217 = Unbundle By Name(w431) -> ("ControlRefs.ProcCore_CtrlQueue"=w492:refnum<queue>)
            n218 = Bundle(cluster=T22 {"queue out"=refnum, "queue out"=refnum}, "queue out"=w491, "queue out"=w473) -> (w482:T22)
            n219 = Initialize Array(w435) -> (w434:T29)  [unwired: 1 in]
            n220 = Bundle By Name(cluster=T23 {"Command"=enum."SetWriterRef", "Params"=variant} ("element"), "Command"=ProcessStates."SetWriterRef", "Params"=w482) -> (w500:T23)
            n221 = Enqueue Element "Set Data queue"(queue=w492, element=w500, error in (no error)=w490) -> (queue out=w485:refnum<queue>, error out=w475:errorcluster)  [unwired: 1 in, 1 out]
            n222 = Dequeue Element(queue=w473, error in (no error)=w475) -> (error out=w474:errorcluster)  [unwired: 1 in, 3 out]
            n223 = Bundle By Name(cluster=T23 {"Command"=enum."SetWriterRef", "Params"=variant} ("element"), "Command"=ProcessStates."StartSave") -> (w487:T23)
            n224 = Unbundle By Name(w467) -> ("Binning.BinWidth"=w463:dbl, "Binning.Minimum"=w464:dbl, "m/z_Array"=w465:dbl[], "Binning.BinType"=w466:T1)
            n225 = Enqueue Element "Start Send Data"(queue=w485, element=w487, error in (no error)=w474) -> (error out=w484:errorcluster)  [unwired: 1 in, 2 out]
            n226 = Unbundle By Name(w467) -> ("File Header.Dimension"=w479:i32[])
            n227 = call <vilib>:"Clear Errors.vi"("error in (no error)"=w484) -> ()  [unwired: 6 in, 1 out]
            n228 = Bundle By Name(cluster=w467, "Binning.Maximum"="MaxiMass", "Binning.Enable"="EnableBinning", "file path"=w448, "file refnum"=w446) -> (w470:T11)
            n229 = Index Array(array=w479) -> (element #1=w478:i32, element #2=w477:i32)  [unwired: 2 in]
            n230 = call "SpectrumBinning_NoGraph.vi"("XScale.Maximum"="MaxiMass", "BinType"=w466, "BinWidth"=w463, "Enable"="EnableBinning", "Signal"=w465, "m/z Array"=w465, "XScale.Minimum"=w464) -> ("m/z Array"=w462:dbl[])  [unwired: 2 in, 2 out]
            n231 = Initialize Array "<= Potential Insufficient Memory Source"(sgl -1.0, w478, w477, 32 ("dimension size")) -> (w481:sgl[][][])
            n232 = Unbundle By Name(w450) -> ("status"=w452:bool)
            n233 = Array Size(array=w462) -> (size(s)=w461:i32)
            n234 = Bundle By Name(cluster=w470, "File Header.SpecLength"=w461, "m/z_Array"=w462) -> (w468:T11)
            n235 = Not(x=w452) -> (.not. x?=w445:bool)
            n236 = call "WriteHeader+MzArray(AnalyzeV75).vi"("error in (no error)"=w450, "ImageConvParams"=w468) -> ("error out"=w469:errorcluster)  [unwired: 9 in]
            n237 = Bundle By Name(cluster=w431, "Save?"=w445) -> (w502:T16)
          }
          frame "PrepScanParams" {
            n238 = Increment(x=w522) -> (x+1=w521:T3)
            n239 = Bundle By Name(cluster=w524, "State"=w521) -> (w523:T15)
            n240 = Unbundle By Name(w536) -> ("Scan#"=w528:i32)
            n241 = Enqueue Element(queue=w525, element=w523) -> ()  [unwired: 2 in, 3 out]
            n242 = Equal To 0?(x=w528) -> (x = 0?=w537:bool)
            n243 = case shown="False" w537 {
              tunnel: w536 -> [w549 w575]
              tunnel: [w539 w571] -> w533
              tunnel: [w543 w574] -> w532
              tunnel: [w542 w573] -> w531
              tunnel: [w541 w572] -> w530
              tunnel: w528 -> [_ w556]
              tunnel: w516 -> [_ _]
              frame True {
                w538 = 0
                # "Initial scan, stick to orignal parameter"
                n244 = Unbundle By Name(w549) -> ("HighSpeed"=w542:dbl, "ScanSpeed"=w541:dbl, "File Header"=w544:T12)
                n245 = Unbundle By Name(w544) -> ("Start Position"=w539:dbl[], "StepWidth"=w547:dbl[], "Dimension"=w548:i32[])
                n246 = Index Array(array=w547, index=w538) -> (element=w546:dbl)
                n247 = Index Array(array=w548, index=w538) -> (element=w545:i32)
                n248 = Multiply(x=w546, y=w545) -> (x*y=w540:dbl)
                n249 = in-place {
                  in-place-border: w540 -> [w551]
                  n250 = in-place-array #4(w539, w538) -> (w552:dbl)
                  n251 = Add(x=w552, y=w551) -> (x+y=w550:dbl)
                  n252 = in-place-array #4(w550) -> (w543:dbl[])  [unwired: 1 out]
                }
              }
              frame False {
                w553 = 1
                w562 = 0 ("index")
                n253 = Unbundle By Name(w575) -> ("HighSpeed"=w573:dbl, "ScanSpeed"=w572:dbl, "File Header"=w564:T12)
                n254 = Unbundle By Name(w564) -> ("Start Position"=w557:dbl[], "StepWidth"=w569:dbl[], "Dimension"=w570:i32[])
                n255 = Index Array(array=w557, index #1=w562, index #2=w553) -> (element #1=w568:dbl, element #2=w559:dbl)
                n256 = Index Array(array=w569, index #1=w562, index #2=w553) -> (element #1=w566:dbl, element #2=w561:dbl)
                n257 = Index Array(array=w570, index #1=w562, index #2=w553) -> (element #1=w565:i32, element #2=w555:i32)
                n258 = Quotient & Remainder "Circle Y #"(x=w556, y=w555) -> (x-y*floor(x/y)=w554:i32)  [unwired: 1 out]
                n259 = Multiply(x=w566, y=w565) -> (x*y=w567:dbl)
                n260 = Multiply(x=w561, y=w554) -> (x*y=w560:dbl)
                n261 = Add "X"(x=w568, y=w567) -> (x+y=w563:dbl)
                n262 = Add "Y"(x=w559, y=w560) -> (x+y=w558:dbl)
                n263 = in-place {
                  in-place-border: w563 -> [w577]
                  in-place-border: w558 -> [w576]
                  # "X"
                  # "Y"
                  n264 = in-place-array #5(w557, w553) -> ()  [unwired: 1 out]
                  n265 = in-place-array #6(w557, w562, w553) -> ()  [unwired: 2 out]
                  n266 = in-place-array #5(w576) -> (w571:dbl[])  [unwired: 1 out]
                  n267 = in-place-array #6(w577, w576) -> (w574:dbl[])  [unwired: 2 out]
                }
              }
            }
            n268 = Bundle By Name(cluster=T26 {"Line Start"=[], "Line End"=[], "HighSpeed"=0.0, "ScanSpeed"=0.0, "KeepStill(ms)"=0, "InstruParams"=[]}, "HighSpeed"=w531, "ScanSpeed"=w530, "Line Start"=w533, "Line End"=w532, "KeepStill(ms)"=u32 0 ("Wait(ms)")) -> (w526:T26)
            n269 = Increment(x=w528) -> (x+1=w535:i32)
            n270 = Enqueue Element "Send scan params"(queue=w527, element=w526) -> (error out=w519:errorcluster)  [unwired: 2 in, 2 out]
            n271 = Bundle By Name(cluster=w536, "Scan#"=w535) -> (w518:T16)
            n272 = Merge Errors(w519, w515) -> (w514:errorcluster)
            n273 = call <vilib>:"Clear Errors.vi"("error in (no error)"=w519) -> ()  [unwired: 6 in, 1 out]
          }
          frame "WaitData" {
            w601 = u32 73  # A prime number to avoid artifact
            # "Only for file conversion\nNothing to do with online conversion"
            # "Potential dead lock"
            # "Need EOF detection, \nAnd set Y Dimension to current value"
            n274 = Dequeue Element "WaitSpectra"(queue=w594) -> (element=w615:T24)  [unwired: 2 in, 3 out]
            n275 = Unbundle By Name(w615) -> ("TickCount"=w588:dbl, "Position"=w599:dbl[], "Spectrum"=w592:sgl[], "Average#"=w590:i32, "Comment"=w585:string)
            n276 = Search and Replace String(input string=w585, search string="EOF" ("y")) -> (number of replacements=w583:i32)  [unwired: 6 in, 3 out]
            n277 = String Subset(string=w585, length (rest)=2 ("length (rest)")) -> (substring=w589:string)  [unwired: 1 in]
            n278 = Type Cast(type=ProcessStates."StartOfLine", x=w589) -> (*(type *) &x=w596:T9)
            n279 = Unbundle By Name(w581) -> ("File Header.Start Position"=w597:dbl[], "File Header.StepWidth"=w598:dbl[])
            n280 = Greater Than 0?(x=w583) -> (x > 0?=w582:bool)
            n281 = Select(t=ProcessStates."Quit", s=w582, f=w596) -> (s? t:f=w587:T9)
            n282 = feedback-in #7(w587) -> ()
            n283 = feedback #7() -> (w595:T9)
            n284 = Multiply(x=w592, y=w590) -> (x*y=w591:sgl[])
            n285 = case "Average Spectra in a single pixel" shown="Default" w587 {
              tunnel: w613 -> [w635 w652 w664 w694]
              tunnel: w610 -> [w622 w649 w662 w692]
              tunnel: w612 -> [_ _ w663 w693]
              tunnel: w606 -> [w632 w648 _ w665]
              tunnel: [_ _ _ w691] -> w607
              tunnel: [w631 w647 _ w690] -> w600
              tunnel: w591 -> [_ _ _ w677]
              tunnel: w599 -> [_ _ _ w676]
              tunnel: w598 -> [_ _ _ w675]
              tunnel: w597 -> [_ _ _ w674]
              tunnel: w595 -> [_ _ _ w672]
              tunnel: [_ _ _ w670] -> _
              tunnel: w590 -> [_ _ _ w667]
              tunnel: w588 -> [_ _ _ _]
              tunnel: [w623 w641 w658 w666] -> w580
              tunnel: w579 -> [w623 w640 w658 w666]
              frame "EndOfLine" {
                # "for debug"
                # "End of Line"
                n286 = Unbundle By Name(w632) -> ("Average"=w633:i32, "Spectra"=w634:sgl[])
                n287 = Enqueue Element At Opposite End(queue=w635, element=T15 {"State"=enum."Flush", "Para."=variant}) -> ()  [unwired: 2 in, 3 out]
                n288 = To Single Precision Float(number=w634) -> (single precision float=w630:sgl[])
                n289 = To Single Precision Float(number=w633) -> (single precision float=w629:sgl)
                n290 = Divide(x=w630, y=w629) -> (x/y=w631:sgl[])
                n291 = Bundle By Name(cluster=w632, "Average"=w633, "Spectra"=w631) -> (w628:T10)
                n292 = Enqueue Element(queue=w622, element=w628) -> ()  [unwired: 2 in, 3 out]
                n293 = feedback #8(0) -> (w625:i32)
                n294 = Increment(x=w625) -> (x+1=w624:i32)
                "#EOL" <- w624
                n295 = feedback-in #8(w624) -> ()
              }
              frame "Quit" {
                # "Does NOT handle 3D image !!"
                # "For incomplete files"
                # "End of File detected (Only for incomplete file)"
                n296 = Unbundle By Name(w648) -> ("Average"=w650:i32, "Spectra"=w651:sgl[])
                n297 = disable-structure shown="Enabled" {
                  disable-tunnel: w652 -> [w656 w657]
                  disable-tunnel: [w655 w657] -> w642
                  frame Disabled {
                    n298 = Enqueue Element At Opposite End(queue=w656, element=T15 {"State"=enum."Close", "Para."=variant}) -> (queue out=w655:refnum<queue>)  [unwired: 2 in, 2 out]
                  }
                  frame Enabled {
                  }
                }
                n299 = To Single Precision Float(number=w651) -> (single precision float=w646:sgl[])
                n300 = To Single Precision Float(number=w650) -> (single precision float=w645:sgl)
                n301 = Unbundle By Name(w640) -> ("File Header.Dimension"=w639:i32[], "Scan#"=w636:i32)
                n302 = Divide(x=w646, y=w645) -> (x/y=w647:sgl[])
                n303 = Bundle By Name(cluster=w648, "Average"=w650, "Spectra"=w647) -> (w644:T10)
                n304 = Enqueue Element(queue=w649, element=w644) -> ()  [unwired: 2 in, 3 out]
                n305 = in-place {
                  in-place-border: w636 -> [w653]
                  n306 = in-place-array #9(w639, 1) -> ()  [unwired: 1 out]
                  n307 = in-place-array #9(w653) -> (w638:i32[])  [unwired: 1 out]
                }
                n308 = Enqueue Element At Opposite End(queue=w642, element=T15 {"State"=enum."Flush", "Para."=variant}) -> ()  [unwired: 2 in, 3 out]
                n309 = Bundle By Name(cluster=w640, "File Header.Dimension"=w638) -> (w641:T16)
              }
              frame "StartOfLine" {
                # "New Line"
                n310 = Enqueue Element "Implied \"WaitData\""(queue=w664, element=w663) -> ()  [unwired: 2 in, 3 out]
                n311 = Flush Queue(queue=w662) -> ()  [unwired: 1 in, 3 out]
                n312 = feedback #10(0) -> (w660:i32)
                n313 = Increment(x=w660) -> (x+1=w659:i32)
                "#SOL" <- w659
                n314 = feedback-in #10(w659) -> ()
              }
              frame Default {
                # "cluster initialize?"
                # "Legacy"
                # "Normal Spectra"
                n315 = Index Array(array=w674) -> (element #1=w685:dbl, element #2=w686:dbl)  [unwired: 2 in]
                n316 = Index Array(array=w675) -> (element #1=w687:dbl, element #2=w688:dbl)  [unwired: 2 in]
                n317 = Index Array(array=w676) -> (element #1=w671:dbl, element #2=w689:dbl)  [unwired: 2 in]
                n318 = Enqueue Element "\"WaitData\" \nImplied"(queue=w694, element=w693) -> ()  [unwired: 2 in, 3 out]
                n319 = Subtract "Y"(x=w689, y=w686) -> (x-y=w682:dbl)
                n320 = Subtract "X"(x=w671, y=w685) -> (x-y=w683:dbl)
                n321 = Divide(x=w682, y=w688) -> (x/y=w681:dbl)
                n322 = Divide(x=w683, y=w687) -> (x/y=w684:dbl)
                n323 = Round Toward -Infinity(1:w684) -> (0:w679:dbl)
                n324 = Round Toward -Infinity(1:w681) -> (0:w680:dbl)
                n325 = To Long Integer(number=w679) -> (32bit integer=w668:i32)
                n326 = To Long Integer(number=w680) -> (32bit integer=w669:i32)
                n327 = call-poly <userlib>:"Data Changed__ogtk.vi"("I32"=w669) -> ("Changed"=w670:bool)
                n328 = Bundle By Name(cluster=w665, "X (Img)"=w668, "Y (Img)"=w669, "Spectra"=w677, "Average"=w667) -> (w678:T10)
                n329 = call-poly <userlib>:"Data Changed__ogtk.vi"("I32"=w668) -> ("Changed"=w673:bool)
                n330 = case shown="False" w673 {
                  tunnel: w692 -> [_ w715]
                  tunnel: w665 -> [w699 w711]
                  tunnel: [w700 w713] -> w691
                  tunnel: w678 -> [w698 w713]
                  tunnel: [w697 w710] -> w690
                  tunnel: w672 -> [_ w708]
                  frame False {
                    # "To be averaged"
                    n331 = Unbundle By Name(w698) -> ("Spectra"=w695:sgl[], "Average"=w696:i32)
                    n332 = in-place {
                      in-place-border: w695 -> [w706]
                      in-place-border: w696 -> [w704]
                      in-place-border: [w703] -> w697
                      n333 = in-place-cluster #11(w699) -> ("Spectra"=w702:sgl[], "Average"=w701:i32)
                      n334 = Compound Arithmetic op=ADD(w702, w706) -> (w703:sgl[])
                      n335 = Compound Arithmetic op=ADD(w701, w704) -> (w705:i32)
                      n336 = in-place-cluster #11("Spectra"=w703, "Average"=w705) -> (w700:T10)
                    }
                  }
                  frame True {
                    # "First one of a pixel"
                    n337 = Unbundle By Name(w711) -> ("Average"=w712:i32, "Spectra"=w716:sgl[])
                    "# average" <- w712
                    n338 = Not Equal?(x=ProcessStates."StartOfLine", y=w708) -> (x != y?=w707:bool)
                    n339 = To Single Precision Float(number=w716) -> (single precision float=w718:sgl[])
                    n340 = To Single Precision Float(number=w712) -> (single precision float=w717:sgl)
                    n341 = Divide(x=w718, y=w717) -> (x/y=w710:sgl[])
                    n342 = Bundle By Name(cluster=w711, "Average"=w712, "Spectra"=w710) -> (w714:T10)
                    n343 = case shown="True" w707 {
                      tunnel: w715 -> [_ w720]
                      tunnel: w714 -> [_ w719]
                      frame False {
                      }
                      frame True {
                        n344 = Enqueue Element ("Push previous to stack")(queue=w720, element=w719) -> ()  [unwired: 2 in, 3 out]
                      }
                    }
                  }
                }
              }
            }
            n345 = Tick Count (ms)() -> (millisecond timer value=w602:u32)
            n346 = Less?(x=w601, y=w602) -> (x < y?=w603:bool)
            n347 = feedback #12() -> (w604:u32)
            n348 = case "raw MS refresh" shown="True" w603 {
              tunnel: w600 -> [_ w620]
              tunnel: w602 -> [_ w621]
              tunnel: [w616 w621] -> w605
              tunnel: w604 -> [w616 _]
              tunnel: w581 -> [_ w618]
              frame False {
              }
              frame True {
                n349 = Unbundle By Name(w618) -> ("m/z_Array"=w619:dbl[])
                n350 = Bundle("m/z_Array"=w619, w620) -> (→"MS (Raw)":cluster{"m/z_Array":dbl[], sgl[]})  [unwired: 1 in]
              }
            }
            n351 = feedback-in #12(w605) -> ()
          }
          frame "Flush" {
            # "Need to be re-written"
            n352 = Preview Queue Element(queue=w761, timeout in ms (-1)=0) -> (queue out=w747:refnum<queue>, element=w744:T15, timed out?=w739:bool, error out=w746:errorcluster)  [unwired: 1 in]
            n353 = Not Equal?(x=T15 {"State"=enum."Close", "Para."=variant}, y=w744) -> (x != y?=w743:cluster{"State":bool, "Para.":bool})
            n354 = Unbundle By Name(w743) -> ("State"=w742:bool)
            n355 = Or(x=w742, y=w739) -> (x .or. y?=w740:bool)
            n356 = case shown="False" w740 {
              tunnel: w760 -> [_ w797]
              tunnel: w759 -> [_ w796]
              tunnel: [w791 w795] -> w754
              tunnel: [w790 w794] -> w753
              tunnel: w747 -> [w791 w793]
              tunnel: w746 -> [w790 w792]
              frame False {
              }
              frame True {
                n357 = Increment(x=w796) -> (x+1=w798:T3)
                n358 = Bundle By Name(cluster=w797, "State"=w798) -> (w799:T15)
                n359 = Enqueue Element(queue=w793, element=w799, error in (no error)=w792) -> (queue out=w795:refnum<queue>, error out=w794:errorcluster)  [unwired: 1 in, 1 out]
              }
            }
            n360 = property on="PeakOI #" class="DigNum (strict)"() -> ("Value"=w750:i32)  [unwired: 2 in, 2 out]
            n361 = Unbundle By Name(w726) -> ("Binning.Maximum"=w731:dbl, "Binning.BinWidth"=w730:dbl, "Binning.Enable"=w724:bool, "Binning.Minimum"=w729:dbl, "m/z_Array"=w725:dbl[], "Binning.BinType"=w728:T1)
            n362 = Unbundle By Name(w738) -> ("InfoBarRef."=w737:refnum<vi>)
            n363 = Bundle By Name(cluster=T15 {"State"=enum."Refresh_Image", "Para."=variant} ("element"), "Para."=w750) -> (w751:T15)
            n364 = Enqueue Element(queue=w754, element=w751, error in (no error)=w753) -> (error out=w723:errorcluster)  [unwired: 1 in, 2 out]
            n365 = Get Queue Status(queue=w727, error in (no error)=w723) -> (queue out=w732:refnum<queue>, # elements in queue=w733:i32)  [unwired: 1 in, 6 out]
            n366 = property class="Str"(reference=w737, error in=w723, "Value"="Flushing: Don't Panic. ") -> (reference out=w736:refnum<vi>)  [unwired: 1 out]
            n367 = case "Batch Binning" shown="True" w724 {
              selector: w724 -> [_ w766]
              tunnel: w733 -> [_ w774]
              tunnel: w732 -> [w764 w773]
              tunnel: w731 -> [_ w772]
              tunnel: w730 -> [_ w771]
              tunnel: w729 -> [_ w770]
              tunnel: w728 -> [_ w769]
              tunnel: [w764 w768] -> _
              tunnel: w725 -> [w762 w767]
              tunnel: [w763 w765] -> w722
              frame False {
                n368 = Array Size(array=w762) -> (size(s)=w763:i32)
              }
              frame True {
                n369 = for {
                  N: w774 -> [_]
                  shift-right: [w783] -> w768
                  shift-left: w773 -> [w789]
                  tunnel: w772 -> [w788]
                  tunnel: w771 -> [w787]
                  tunnel: w766 -> [w786]
                  tunnel: w770 -> [w785]
                  tunnel: w769 -> [w784]
                  tunnel: w767 -> [w778]
                  tunnel: [w775] -> w765
                  n370 = Dequeue Element(queue=w789) -> (queue out=w782:refnum<queue>, element=w781:T10)  [unwired: 2 in, 2 out]
                  n371 = Unbundle By Name(w781) -> ("Spectra"=w779:sgl[])
                  n372 = call "SpectrumBinning_NoGraph.vi"("XScale.Maximum"=w788, "BinType"=w784, "BinWidth"=w787, "Enable"=w786, "Signal"=w779, "m/z Array"=w778, "XScale.Minimum"=w785) -> ("Spectrum"=w777:dbl[], "m/z Array"=w776:dbl[])  [unwired: 2 in, 1 out]
                  n373 = Bundle By Name(cluster=w781, "Spectra"=w777) -> (w780:T10)
                  n374 = Array Size(array=w776) -> (size(s)=w775:i32)
                  n375 = Enqueue Element(queue=w782, element=w780) -> (queue out=w783:refnum<queue>)  [unwired: 2 in, 2 out]
                }
              }
            }
            n376 = Increment(x=w748) -> (x+1=w749:i32)
            n377 = Bundle By Name(cluster=w726, "File Header.SpecLength"=w722) -> ()  [unwired: 1 out]
            n378 = call <vilib>:"General Error Handler.vi"() -> ("error out"=w755:errorcluster)  [unwired: 11 in, 4 out]
            n379 = property class="Str"(reference=w736, "Value"="") -> ()  [unwired: 1 in, 2 out]
            "Line#" <- w748
          }
          frame "ScanResult" {
            # "For comapatibility with other static subprogram, drive the loop going"
            n380 = Increment(x=w807) -> (x+1=w810:T3)
            n381 = Bundle By Name(cluster=w808, "State"=w810) -> (w811:T15)
            n382 = Enqueue Element(queue=w809, element=w811) -> ()  [unwired: 2 in, 3 out]
          }
          frame "CheckEndCondition" {
            w828 = 2  # axis:Z
            w835 = 1  # axis:Y
            # "Some bug may exist"
            # "fitted for 3D imaing, \nmay not fit for binary file conversion"
            # "Add condition:\nreader quit due to file ends"
            n383 = Unbundle By Name(w820) -> ("Scan#"=w826:i32, "File Header.Dimension"=w836:i32[])
            n384 = Index Array(array=w836, index #1=w835, index #2=w828) -> (element #1=w825:i32, element #2=w817:i32)
            n385 = Multiply(x=w825, y=w817) -> (x*y=w827:i32)
            n386 = Quotient & Remainder(x=w826, y=w825) -> (x-y*floor(x/y)=w818:i32, floor(x/y)=w816:i32)
            n387 = Subtract(x=w827, y=w826) -> (x-y=→"remaining lines":i32)
            n388 = Equal To 0? "2D_Image finished?"(x=w818) -> (x = 0?=w815:bool)
            n389 = Greater Or Equal? "3D_Image finished"(x=w816, y=w817) -> (x >= y?=w814:bool)
            n390 = case "One Image Finish" shown="True" w815 {
              tunnel: w816 -> [_ w840]
              tunnel: [T15 {"State"=enum."PrepScanParams", "Para."=variant} w850] -> w823
              tunnel: w822 -> [w838 w856]
              tunnel: [w838 w855] -> w821
              tunnel: w819 -> [_ w853]
              frame False {
                # "Continue next line scan"
              }
              frame True {
                # "If the file exist, error will be thrown out \nand will crash the expt !, proper error handling needed"
                # "to be done"
                # "A signal image finished in 3D imaging."
                n391 = Unbundle By Name(w853) -> ("file path"=w851:path)
                n392 = Enqueue Element(queue=w856, element=T15 {"State"=enum."Close", "Para."=variant}) -> (queue out=w855:refnum<queue>)  [unwired: 2 in, 2 out]
                n393 = Strip Path(path=w851) -> (stripped path=w852:path, name=w841:string)
                n394 = Format Value(string ("")="_", format string="%04d", value (0)=w840) -> (output string=w846:string)
                n395 = xnode "Match Regular Expression"("input string"=w841, "regular expression"="((_[0-9]+)?)(\\..[^.]*$)") -> ("before match"=w848:string, "submatch 3"=w843:string)  [unwired: 4 in, 6 out]
                n396 = Concatenate Strings "Append depth number"(w848, w846, w843) -> (w842:string)
                n397 = Build Path(base path=w852, name or relative path=w842) -> (appended path=w849:path)
                n398 = Bundle By Name(cluster=T15 {"State"=enum."Open", "Para."=variant}, "Para."=w849) -> (w850:T15)
              }
            }
            n399 = Select(t=T15 {"State"=enum."Close", "Para."=variant}, s=w814, f=w823) -> (s? t:f=w829:T15)
            n400 = Enqueue Element(queue=w821, element=w829) -> ()  [unwired: 2 in, 3 out]
          }
          frame "Close" {
            # "need to reset registers?\n\nNo"
            n401 = Unbundle By Name(w980) -> ("file refnum"=w981:refnum<file>)
            n402 = Close File(refnum=w981, error in=w978) -> (error out=w977:errorcluster)  [unwired: 1 out]
            n403 = call <vilib>:"Clear Errors.vi"("error in (no error)"=w977) -> ()  [unwired: 6 in, 1 out]
            n404 = Unbundle By Name(w994) -> ("ControlRefs.ProcCore_CtrlQueue"=w989:refnum<queue>, "ControlRefs.WriterSIG"=w993:refnum<queue>)
            n405 = property on="Cancel" class="Bool"("Visible"=FALSE) -> ()  [unwired: 2 in, 2 out]
            n406 = property on="Close/Quit" class="Bool (strict)"("BoolText.Text"="Done" ("Boolean Text.Text")) -> ()  [unwired: 2 in, 2 out]
            n407 = Bundle By Name(cluster=T23 {"Command"=enum."SetWriterRef", "Params"=variant} ("element"), "Command"=ProcessStates."StopSave") -> (w988:T23)
            n408 = Bundle By Name(cluster=T23 {"Command"=enum."SetWriterRef", "Params"=variant} ("element"), "Command"=ProcessStates."SetWriterRef", "Params"=w993) -> (w996:T23)
            n409 = Enqueue Element(queue=w989, element=w988) -> (queue out=w987:refnum<queue>, error out=w986:errorcluster)  [unwired: 2 in, 1 out]
            n410 = Enqueue Element(queue=w987, element=w996, error in (no error)=w986) -> (error out=w985:errorcluster)  [unwired: 1 in, 2 out]
            n411 = call <vilib>:"Clear Errors.vi"("error in (no error)"=w985) -> ()  [unwired: 6 in, 1 out]
          }
          frame "Quit" {
            n412 = disable-structure shown="Enabled" {
              disable-tunnel: w1005 -> [w1019 _]
              frame Enabled {
                # "maybe not needed anymore, needed to be tested!!"
                # "Bad solution: have upper level jump out wait queue"
                n413 = Enqueue Element(queue=w1019, element=T26 {"Line Start"=[], "Line End"=[], "HighSpeed"=0.0, "ScanSpeed"=0.0, "KeepStill(ms)"=0, "InstruParams"=[]}) -> (error out=w1017:errorcluster)  [unwired: 2 in, 2 out]
                n414 = call <vilib>:"Clear Errors.vi"("error in (no error)"=w1017) -> ()  [unwired: 6 in, 1 out]
              }
              frame Disabled {
              }
            }
            n415 = Release Queue(queue=w1013, error in (no error)=w1000) -> (error out=w1002:errorcluster)  [unwired: 1 in, 2 out]
            n416 = Generate User Event(user event=w1010, event data cluster=cluster{bool} {TRUE} ("event data")) -> (user event out=w1008:refnum<user-event>, error out=w1007:errorcluster)  [unwired: 2 in]
            n417 = Destroy User Event(user event=w1008, error in=w1007) -> (error out=w1006:errorcluster)
            n418 = Merge Errors(w1006, w1002) -> (w1001:errorcluster)
          }
          frame "Refresh_Image" {
            w1033 = 0.0 ("Z Scale.Range:Minimum")
            # "Call command has to be push to the end not start of the queue."
            n419 = Unbundle By Name(w1038) -> ("Para."=w1037:variant)
            n420 = Variant To Data(type=1 ("PeakOI #"), Variant=w1037) -> (data=w1034:i32)  [unwired: 1 in, 1 out]
            n421 = Array Subset(array=w1041, index (dim 2)=w1034, length (dim 2)=1 ("length")) -> (w1040:sgl[][][])  [unwired: 4 in]
            n422 = control-ref of="ImagePreview"() -> (w1022:refnum<vi>)
            n423 = Array Size(array=w1040) -> (size(s)=w1039:i32[])
            n424 = Index Array(array=w1039) -> (element #1=w1032:i32, element #2=w1031:i32)  [unwired: 3 in, 1 out]
            n425 = Max & Min(x=w1032, y=w1031) -> (max(x,y)=w1030:i32)  [unwired: 1 out]
            n426 = Reshape Array(w1040, w1032, w1031) -> (w1021:sgl[][])
            n427 = property on="Fix race condition \n(autoscale related)" class="IntGraph (strict)"(reference=w1022, "Value"=w1021) -> (reference out=w1023:refnum<vi>, error out=w1024:errorcluster)  [unwired: 1 in]
            n428 = property class="IntGraph (strict)"(reference=w1023, error in=w1024) -> (reference out=w1029:refnum<vi>, "ZScale.Maximum"=w1026:dbl)  [unwired: 1 out]
            n429 = Array Max & Min(array=w1021) -> (max value=w1028:sgl)  [unwired: 3 out]
            n430 = Select(t=w1028, s="AutoScaleZ", f=w1026) -> (s? t:f=w1027:dbl)
            n431 = property class="IntGraph (strict)"(reference=w1029, "ZScale.Maximum"=w1027, "ZScale.Minimum"=w1033, "XScale.Minimum"=w1033, "XScale.Maximum"=w1030, "YScale.Minimum"=w1033, "YScale.Maximum"=w1030) -> ()  [unwired: 1 in, 2 out]
          }
          frame "Refresh_Profile" {
            n432 = Unbundle By Name(w1049) -> ("mzArray"=w1048:dbl[])
            n433 = Subtract(x="m/z (Da)", y="Integration Width (±Da)") -> (x-y=w1055:dbl)
            n434 = Add(x="m/z (Da)", y="Integration Width (±Da)") -> (x+y=w1054:dbl)
            n435 = Threshold 1D Array(2:w1055, 3:w1048) -> (0:w1058:dbl)  [unwired: 1 in]
            n436 = Round Toward -Infinity(1:w1058) -> (0:w1056:dbl)
            n437 = Threshold 1D Array(1:w1056, 2:w1054, 3:w1048) -> (0:w1057:dbl)
            n438 = for {
              tunnel: w1051 -> [w1071] mode=indexing
              tunnel: [w1067] -> w1050 mode=indexing
              tunnel: w1057 -> [w1066]
              tunnel: w1056 -> [w1065]
              n439 = Unbundle By Name(w1071) -> ("Spectra"=w1070:sgl[])
              n440 = Subtract(x=w1066, y=w1065) -> (x-y=w1069:dbl)
              n441 = Array Subset(array=w1070, index=w1065, length=w1069) -> (w1068:sgl[])
              n442 = call-poly <vilib>:"Mean.vi"("X"=w1068) -> ("mean"=w1067:dbl)  [unwired: 1 out]
            }
            "Depth Profile" <- w1050
          }
          frame "Refresh_Spectra" {
            n443 = Decrement(x="Shot#") -> (x-1=w1081:i32)
            n444 = for {
              N: "#Layers" -> [_]
              tunnel: w1079 -> [w1101]
              tunnel: w1081 -> [w1099]
              shift-right: [w1097] -> w1085
              shift-left: _ -> [w1096]
              tunnel: [w1094] -> w1083
              tunnel: [w1093] -> _ mode=indexing
              i -> [w1094]
              n445 = Add(x=w1099, y=w1094) -> (x+y=w1098:i32)
              n446 = Index Array(array=w1101, index=w1098) -> (element=w1100:T10)
              n447 = Unbundle By Name(w1100) -> ("Spectra"=w1093:sgl[])
              n448 = Equal To 0?(x=w1094) -> (x = 0?=w1095:bool)
              n449 = case shown="False" w1095 {
                tunnel: [w1104 w1105] -> w1097
                tunnel: w1096 -> [w1103 _]
                tunnel: w1093 -> [w1102 w1105]
                frame False {
                  n450 = Add(x=w1102, y=w1103) -> (x+y=w1104:sgl[])
                }
                frame True {
                }
              }
            }
            n451 = Unbundle By Name(w1078) -> ("mzArray"=w1086:dbl[])
            n452 = Increment(x=w1083) -> (x+1=w1082:i32)
            n453 = Reciprocal(x=w1082) -> (1/x=w1084:dbl)
            n454 = control-ref of="Spectra"() -> (w1074:refnum<vi>)
            n455 = Multiply(x=w1085, y=w1084) -> (x*y=w1080:dbl[])
            n456 = call-poly "SpecBinning.vi"("BinType"="BinType", "BinWidth"="BinWidth", "Signal"=w1080, "m/z Array"=w1086, "GraphRef."=w1074) -> ("BinnedSpectrum"=→"Spectra":cluster{"m/z Array":dbl[], "Signal":dbl[]})  [unwired: 5 in, 1 out]
          }
          frame "SaveMiddleFile" {
            n457 = call <vilib>:"Dflt Data Dir.vi"() -> ("App:Default Data Directory"=w1117:path)
            n458 = feedback #13(w1117) -> (w1115:path)
            n459 = Strip Path(path=w1115) -> (stripped path=w1111:path, name=w1112:string)
            n460 = call "File Dialog"("start path"=w1111, "default name"=w1112, "pattern (all files)"="*.dp.bin", "pattern label"="Depth Profile File") -> ("selected path"=w1113:path, "cancelled"=w1108:bool, "error out"=w1116:errorcluster)  [unwired: 8 in, 1 out]
            n461 = case shown="False" w1108 {
              tunnel: w1113 -> [w1128 _]
              tunnel: [w1128 w1129] -> w1114
              tunnel: w1115 -> [_ w1129]
              tunnel: w1116 -> [w1127 _]
              tunnel: w1106 -> [w1124 _]
              tunnel: [w1126 _] -> _
              tunnel: w1107 -> [w1125 _]
              frame False {
                n462 = call "DepthProfileFormat_Writer.vi"("error in"=w1127, "DepthProfilingArray"=w1124, "AcquisitionParams."=w1125, "depth profile file path"=w1128) -> ("error out"=w1126:errorcluster)  [unwired: 7 in]
              }
              frame True {
              }
            }
            n463 = feedback-in #13(w1114) -> ()
          }
          frame "Save_Image" {
            # "Call command has to be push to the end not start of the queue."
            n464 = control-ref of="Peaks of Interest"() -> (w1141:refnum<vi>)
            n465 = Unbundle By Name(w1172) -> ("Para."=w1171:variant)
            n466 = property class="Tbl (strict)"(reference=w1141) -> ("Value"=w1140:string[][])  [unwired: 1 in, 2 out]
            n467 = Variant To Data(type=1 ("PeakOI #"), Variant=w1171) -> (data=w1139:i32)  [unwired: 1 in, 1 out]
            n468 = Unbundle By Name(w1132) -> ("file path"=w1131:path)
            n469 = Index Array(array=w1140, index (row) #1=w1139, index (col) #1=0 ("disabled index (col)"), index (row) #2=w1139, index (col) #2=1 ("disabled index (col)")) -> (element #1=w1136:string, element #2=w1135:string)
            n470 = control-ref of="ImagePreview"() -> (w1166:refnum<vi>)
            n471 = Strip Path(path=w1131) -> (stripped path=w1146:path, name=w1150:string)
            n472 = Array Subset(array=w1175, index (dim 2)=w1139, length (dim 2)=1 ("length")) -> (w1174:sgl[][][])  [unwired: 4 in]
            n473 = property class="IntGraph (strict)" props=["Color Table", "ZScale", "Maximum", "ZScale", "Minimum", "XScale", "Minimum", "XScale", "Maximum", "YScale", "Minimum", "YScale", "Maximum"](reference=w1166) -> ("Color Table"=w1143:u32[], "ZScale.Maximum"=w1144:dbl, "ZScale.Minimum"=w1145:dbl)  [unwired: 1 in, 6 out]
            n474 = xnode "Match Regular Expression"("input string"=w1150, "regular expression"="(\\..[^.]*$)") -> ("before match"=w1163:string)  [unwired: 4 in, 4 out]
            n475 = Format Into String(format string="_%s(+-%s)", w1136, w1135) -> (resulting string=w1162:string)  [unwired: 2 in, 1 out]
            n476 = Array Size(array=w1174) -> (size(s)=w1173:i32[])
            n477 = Index Array(array=w1173) -> (element #1=w1168:i32, element #2=w1167:i32)  [unwired: 3 in, 1 out]
            n478 = Concatenate Strings(w1163, w1162, ".png" ("string")) -> (w1147:string)
            n479 = Reshape Array(w1174, w1168, w1167) -> (w1142:sgl[][])
            n480 = Subtract(x=w1144, y=w1145) -> (x-y=w1156:dbl)
            n481 = Build Path(base path=w1146, name or relative path=w1147) -> (appended path=w1148:path)
            n482 = Subtract(x=w1142, y=w1145) -> (x-y=w1165:dbl[][])
            n483 = Divide(x=256.0 ("Img_coeff."), y=w1156) -> (x/y=w1158:dbl)
            n484 = Array Size(array=w1165) -> (size(s)=w1151:i32[])
            n485 = Compound Arithmetic op=MULTIPLY(w1158, w1165) -> (w1159:dbl[][])
            n486 = Transpose 2D Array(2D array=w1159) -> (transposed array=w1160:dbl[][])
            n487 = Index Array(array=w1151) -> (element #1=w1153:i32, element #2=w1154:i32)  [unwired: 2 in]
            n488 = Round Toward -Infinity(1:w1160) -> (0:w1161:dbl[][])
            n489 = Multiply(x=w1153, y=w1154) -> (x*y=w1155:i32)
            n490 = To Unsigned Byte Integer(number=w1161) -> (unsigned 8bit integer=w1152:u8[][])
            n491 = disable-structure shown="Enabled" {
              disable-tunnel: w1143 -> [w1191 _]
              disable-tunnel: w1148 -> [w1190 w1194]
              disable-tunnel: w1152 -> [w1186 w1195]
              disable-tunnel: w1153 -> [w1184 _]
              disable-tunnel: w1154 -> [w1183 _]
              disable-tunnel: w1155 -> [w1182 _]
              frame Enabled {
                n492 = Reshape Array(w1186, w1182) -> (w1185:u8[])
                n493 = Bundle By Name(cluster=T27 {"image type"=0, "image depth"=32, "image"=[], "mask"=[], "colors"=[], "Rectangle"={"left"=0, "top"=0, "right"=256, "bottom"=256}} ("Image Data 2"), "colors"=w1191, "image type"=0, "image depth"=8, "image"=w1185, "Rectangle.right"=w1184, "Rectangle.bottom"=w1183) -> (w1181:T27)
                n494 = call <vilib>:"Write PNG File.vi"("image data"=w1181, "path to PNG file"=w1190) -> ("error out"=w1180:errorcluster)  [unwired: 8 in, 1 out]
                n495 = call <vilib>:"Clear Errors.vi"("error in (no error)"=w1180) -> ()  [unwired: 6 in, 1 out]
              }
              frame Disabled {
                n496 = call "IMAQ ArrayToImage"("Image Pixels (U8)"=w1195) -> ("Image Out"=w1193:T30)  [unwired: 9 in, 1 out]
                n497 = call-poly "IMAQ Write File 2"("TIFF Options"=T28 {"Rows Per Strip"=0, "Photometric"=1, "Compression Type"=3}, "File Path"=w1194, "Image"=w1193) -> ()  [unwired: 7 in, 2 out]
              }
            }
          }
          frame "SetPeakOI" {
            n498 = Unbundle By Name(w1315) -> ("PeakOI"=w1311:cluster{"m/z":dbl, "Width(+/-)":dbl}[])
            n499 = Unbundle By Name(w1317) -> ("Para."=w1316:variant)
            n500 = Variant To Data(type=w1311, Variant=w1316) -> (data=w1313:cluster{"m/z":dbl, "Width(+/-)":dbl}[], error out=w1314:errorcluster)  [unwired: 1 in]
            n501 = Select(t=w1311, s=w1314, f=w1313) -> (s? t:f=w1312:cluster{"m/z":dbl, "Width(+/-)":dbl}[])
            n502 = Bundle By Name(cluster=w1315, "PeakOI"=w1312) -> (w1320:T11)
          }
          frame Default {
          }
        }
        n503 = call <userlib>:"ErrorLog.vi"("error in (no error)"=w376) -> ("error out"=w375:errorcluster)  [unwired: 10 in]
      }
      frame Error {
      }
    }
    "Iteration" <- w349
  }
  n504 = Release Queue "Release Queue\nAfter all quit."(queue=w20, error in (no error)=w22) -> (error out=→"error out":errorcluster)  [unwired: 1 in, 2 out]
  n505 = disable-structure "For legacy files, manually add EOL mark" shown="Disabled" {
    frame Disabled {
      w1340 = FALSE  # True for missing EOL (Legacy)
      n506 = And(y=w1340) -> (x .and. y?=w1339:bool)  [unwired: 1 in]
      n507 = case "For Legacy Code" shown="True" w1339 {
        tunnel: _ -> [_ w1346]
        frame False {
        }
        frame True {
          n508 = Type Cast(type="", x=ProcessStates."EndOfLine") -> (*(type *) &x=w1345:string)
          n509 = Bundle By Name(cluster=T24 {"SampleRate"=-1.0, "TrigDelay"=0.0, "SpecLength"=0.0, "DAQ_Range"=0.0, "Average#"=0, "Position"=[], "Spectrum"=[], "Calibr."=[], "Pressure"=-1.0, "Desp_LaserEnergy"=-1.0, "PI_LaserEnergy"=-1.0, "Voltages Table"=[], "ProcMode"=enum."None", "Threshold"=-1.0, "Comment"="", "TickCount"=0.0, "Time Stamp"=timestamp(0 s since 1904-01-01)} ("Value"), "Comment"=w1345) -> (w1341:T24)
          n510 = Enqueue Element At Opposite End(queue=w1346, element=w1341) -> ()  [unwired: 2 in, 3 out]
        }
      }
    }
    frame Enabled {
    }
  }
